vi "Demo_Main3.vi"() -> ()   [LabVIEW 2010]
uses:
  ControlCAN/ControlCAN.llb/DevType.ctl
  ControlCAN/ControlCAN.llb/CAN Channel.ctl
  ControlCAN/ControlCAN.llb/InitFlag.ctl
  ControlCAN/ControlCAN.llb/Mode.ctl
  ControlCAN/ControlCAN.llb/Fliter.ctl
  ControlCAN/ControlCAN.llb/VCI_CAN_OBJ.ctl
  ControlCAN/ControlCAN.llb/VCI_INIT_CONFIG.ctl
  ControlCAN/ControlCAN.llb/Return Val.ctl
  ControlCAN/ControlCAN.lvlib
panel:
  out "ERRO7":bool
  out "ERRO6":bool
  out "ERRO5":bool
  out "ERRO4":bool
  out "ERRO3":bool
  out "高温":bool
  out "高压":bool
  out "低压":bool
  out "warn7":bool
  out "warn6":bool
  out "warn5":bool
  out "warn4":bool
  out "warn3":bool
  out "高温":bool
  out "warn1":bool
  out "warn0":bool
  out "温度":dbl format="%#.6f"
  out "转速":dbl(graph)
  out "CAN ID":u8 format="%x"
  out "数组":u8[](array[numeric]) format="%x"
  in  "DATA_SAVE_W":bool
  out "CI_K0_回":u16
  out "BI_K0_回":u16
  in  "CI_K0_R":bool
  in  "BI_K0_R":bool
  in  "CI_K0_W":bool
  in  "BI_K0_W":bool
  in  "C电流零偏":u16
  in  "B电流零偏":u16
  in  "AI_K0_R":bool
  in  "A电流零偏":u16
  out "AI_K0_回":u16
  in  "AI_K0_W":bool
  out "Sin":i32
  out "Cosin":i32
  in  "加速度_R":bool
  in  "加速度":dbl min=0.0 max=8000.0 format="%#.6f"
  out "加速度_回":dbl format="%#.6f"
  in  "加速度_W":bool
  in  "速度环KI_R":bool
  in  "速度环KP_R":bool
  in  "速度环KI":dbl format="%#.6f"
  out "速度环KI_回":dbl format="%#.6f"
  in  "速度环KI_W":bool
  in  "速度环KP":dbl format="%#.6f"
  out "速度环KP_回":dbl format="%#.6f"
  in  "速度环KP_W":bool
  in  "电流环KI_R":bool
  in  "电流环KP_R":bool
  in  "电流环KI":dbl format="%#.6f"
  out "电流环KI_回":dbl format="%#.6f"
  in  "电流环KI_W":bool
  in  "电流环KP":dbl format="%#.6f"
  out "电流环KP_回":dbl format="%#.6f"
  in  "电流环KP_W":bool
  out "波形图表3":dbl(graph)
  out "波形图表2":dbl(graph)
  out "波形图表1":dbl(graph)
  out "sCnt":u32 caption="处理统计"
  out "模式_回":string(combo)="00"
  in  "模式_R":bool
  in  "设定电流_R":bool
  in  "设定位置_R":bool
  in  "设定速度_R":bool
  in  "存储路径":path
  in  "保存":bool
  out "保存_S":bool
  in  "模式_W":bool
  in  "模式":string(combo)="00"
  in  "设定电流":dbl format="%#.6f"
  out "设定电流_回":dbl format="%#.6f"
  in  "设定电流_W":bool
  in  "设定位置":dbl format="%#.6f"
  out "设定位置_回":dbl format="%#.6f"
  in  "设定位置_W":bool
  in  "设定速度":dbl format="%#.1f"
  out "设定速度_回":dbl format="%#.6f"
  in  "设定速度_W":bool
  in  "监测_W":bool
  in  "监测":string(combo)="30"
  out "电机ID_R":u32
  in  "Clear":bool
  out "Ualfa":dbl format="%#.6f"
  out "Ubate":dbl format="%#.6f"
  out "Uq":dbl format="%#.6f"
  out "Ud":dbl format="%#.6f"
  out "PWM1":u16
  out "PWM2":u16
  out "PWM3":u16
  out "sector":u8
  out "Iqnow":dbl
  out "Idnow":dbl
  out "Ialfa":dbl
  out "Ibeta":dbl
  out "A电流":dbl
  out "C电流":dbl
  out "B电流":dbl
  out "供电电压":dbl
  out "机械角度":dbl format="%.2f"
  out "电气角度":dbl
  out "转速":dbl
  out "CAN STD_ID":u32 format="%x"
  in  "电机ID":string(combo)="00"
  in  "电机ID_W":bool
  out "RecvCnt":u32 caption="接收统计"
  out "SendCnt":u32 caption="发送统计"
  in  "Format":u8(ring) items=["标准帧", "扩展帧"]
  in  "Type":u8(ring) items=["数据帧", "远程帧"]
  in  "Data":string="00 01 02 03 04 05 06 07"
  in  "ID":u32=291 format="0x%x"
  in  "Send":bool
  in  "RcvEnable":bool=TRUE
  out "Open":bool
  in  "Fliter":T1=1 items=["接收所有类型"=1, "只接收标准帧"=2, "只接收扩展帧"=3]
  in  "kBaudRate":u8(ring)=12 caption="波特率" items=["5k bps"=1, "10k bps"=2, "20k bps"=3, "40k bps"=4, "50k bps"=5, "80k bps"=6, "100k bps"=7, "125k bps"=8, "200k bps"=9, "250k bps"=10, "400k bps"=11, "500k bps"=12, "666k bps"=13, "800k bps"=14, "1000k bps"=15, "33.33k bps"=16, "66.66k bps"=17, "83.33k bps"=18]
  in  "Mode":T2 caption="工作模式" items=["正常工作", "仅侦听模式", "自测模式（环回）"]
  in  "InitFlag":T3 caption="初始化参数" items=["使用Flash参数", "使用界面设置参数"]
  in  "AccMask":u32=4294967295 caption="接收屏蔽码" format="%08x"
  in  "AccCode":u32 caption="接收过滤码" format="%08x"
  in  "Close":bool
  in  "Open":bool
  in  "Channel":T4 caption="CAN通道" items=["通道1", "通道2"]
  in  "DevType":T5=3 caption="设备类型" items=["USB-CAN"=2, "USB-CAN2"=3]
  # "."
  # "发送指令帧包"
  # "CAN\n  ID"
  # "DATA"
  # "DATA"
  # "DATA"
  # "0"
  # "1"
  # "7"
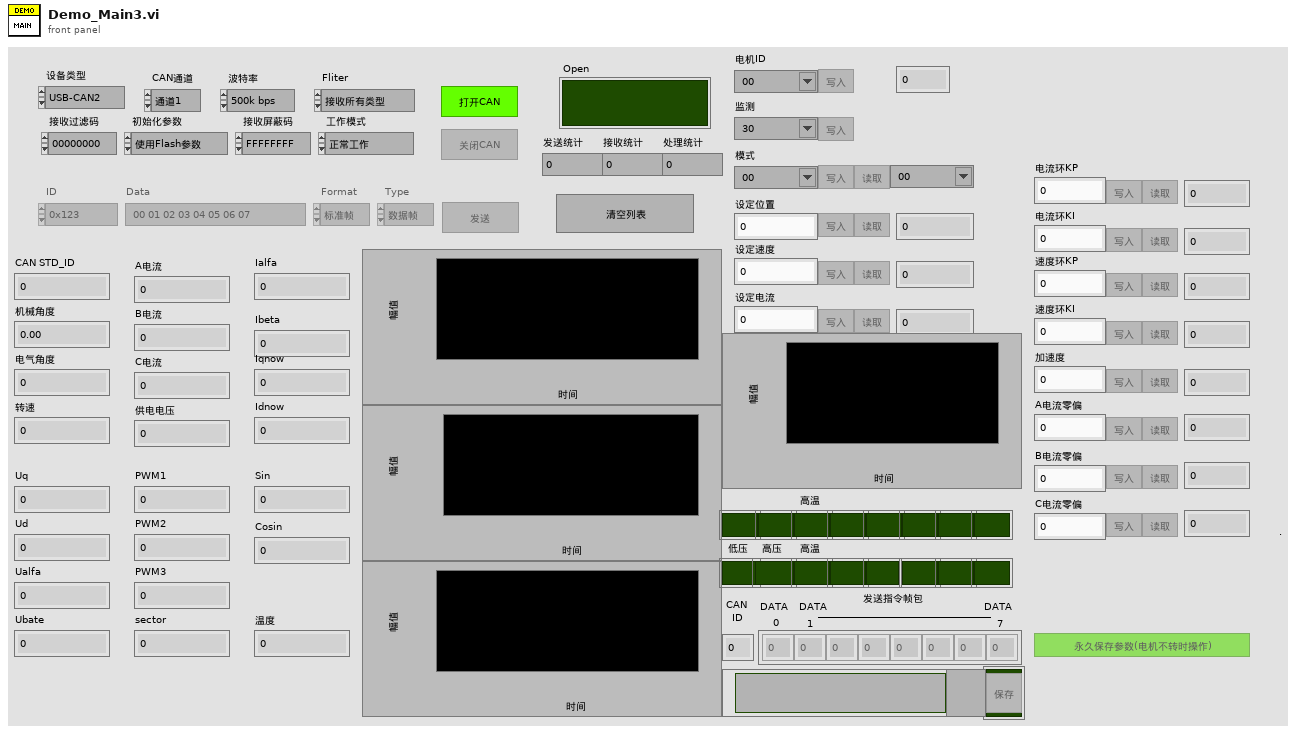
[diagram p1: front panel]
types:
  T1 = typedef "ControlCAN.lvlib/Fliter.ctl" = u8
  T2 = typedef "ControlCAN.lvlib/Mode.ctl" = u8
  T3 = typedef "ControlCAN.lvlib/InitFlag.ctl" = u32
  T4 = typedef "ControlCAN.lvlib/CAN Channel.ctl" = u32
  T5 = typedef "ControlCAN.lvlib/DevType.ctl" = u32
  T6 = typedef "ControlCAN.lvlib/VCI_CAN_OBJ.ctl" = cluster{"ID":u32, "TimeStamp":u32, "TimeFlag":u8, "SendType":u8, "RemoteFlag":u8, "ExternFlag":u8, "DataLen":u8, "Data":u8[], "Reserved":u8[]}
  T7 = cluster{"Type":enum16{"接收", "发送"}, "Channel":T4, "Time":timestamp, "VCI_CAN_OBJ":T6}[]
  T8 = typedef "ControlCAN.lvlib/VCI_INIT_CONFIG.ctl" = cluster{"AccCode":u32, "AccMask":u32, "InitFlag":T3, "Fliter":T1, "Timing0":u8, "Timing1":u8, "Mode":T2}
  T9 = cluster{"DevType":T5, "DevIndex":u32, "CanIndex":T4, "VCI_INIT_CONFIG":T8}
  T10 = typedef "ControlCAN.lvlib/Return Val.ctl" = i32
  T11 = enum16{"open", "replace", "create", "open or create", "replace or create", "replace or create with confirmation"}
  T12 = cluster{"[0]":cluster{"Type":enum16{"接收", "发送"}, "Channel":T4, "Time":timestamp, "VCI_CAN_OBJ":T6}}
  T13 = cluster{"Type":enum16{"接收", "发送"}, "Channel":T4, "Time":timestamp, "VCI_CAN_OBJ":T6}
  T14 = cluster{"Data[0]":u8, "Data[1]":u8, "Data[2]":u8, "Data[3]":u8, "Data[4]":u8, "Data[5]":u8, "Data[6]":u8, "Data[7]":u8}
  T15 = cluster{"Boolean array[0]":bool, "Boolean array[1]":bool, "Boolean array[2]":bool, "Boolean array[3]":bool, "Boolean array[4]":bool, "Boolean array[5]":bool, "Boolean array[6]":bool, "Boolean array[7]":bool}
  T16 = enum32{"invalid app kind", "Development System", "Run Time System", "Student Edition", "Embedded LabVIEW", "Evaluation", "Custom"}
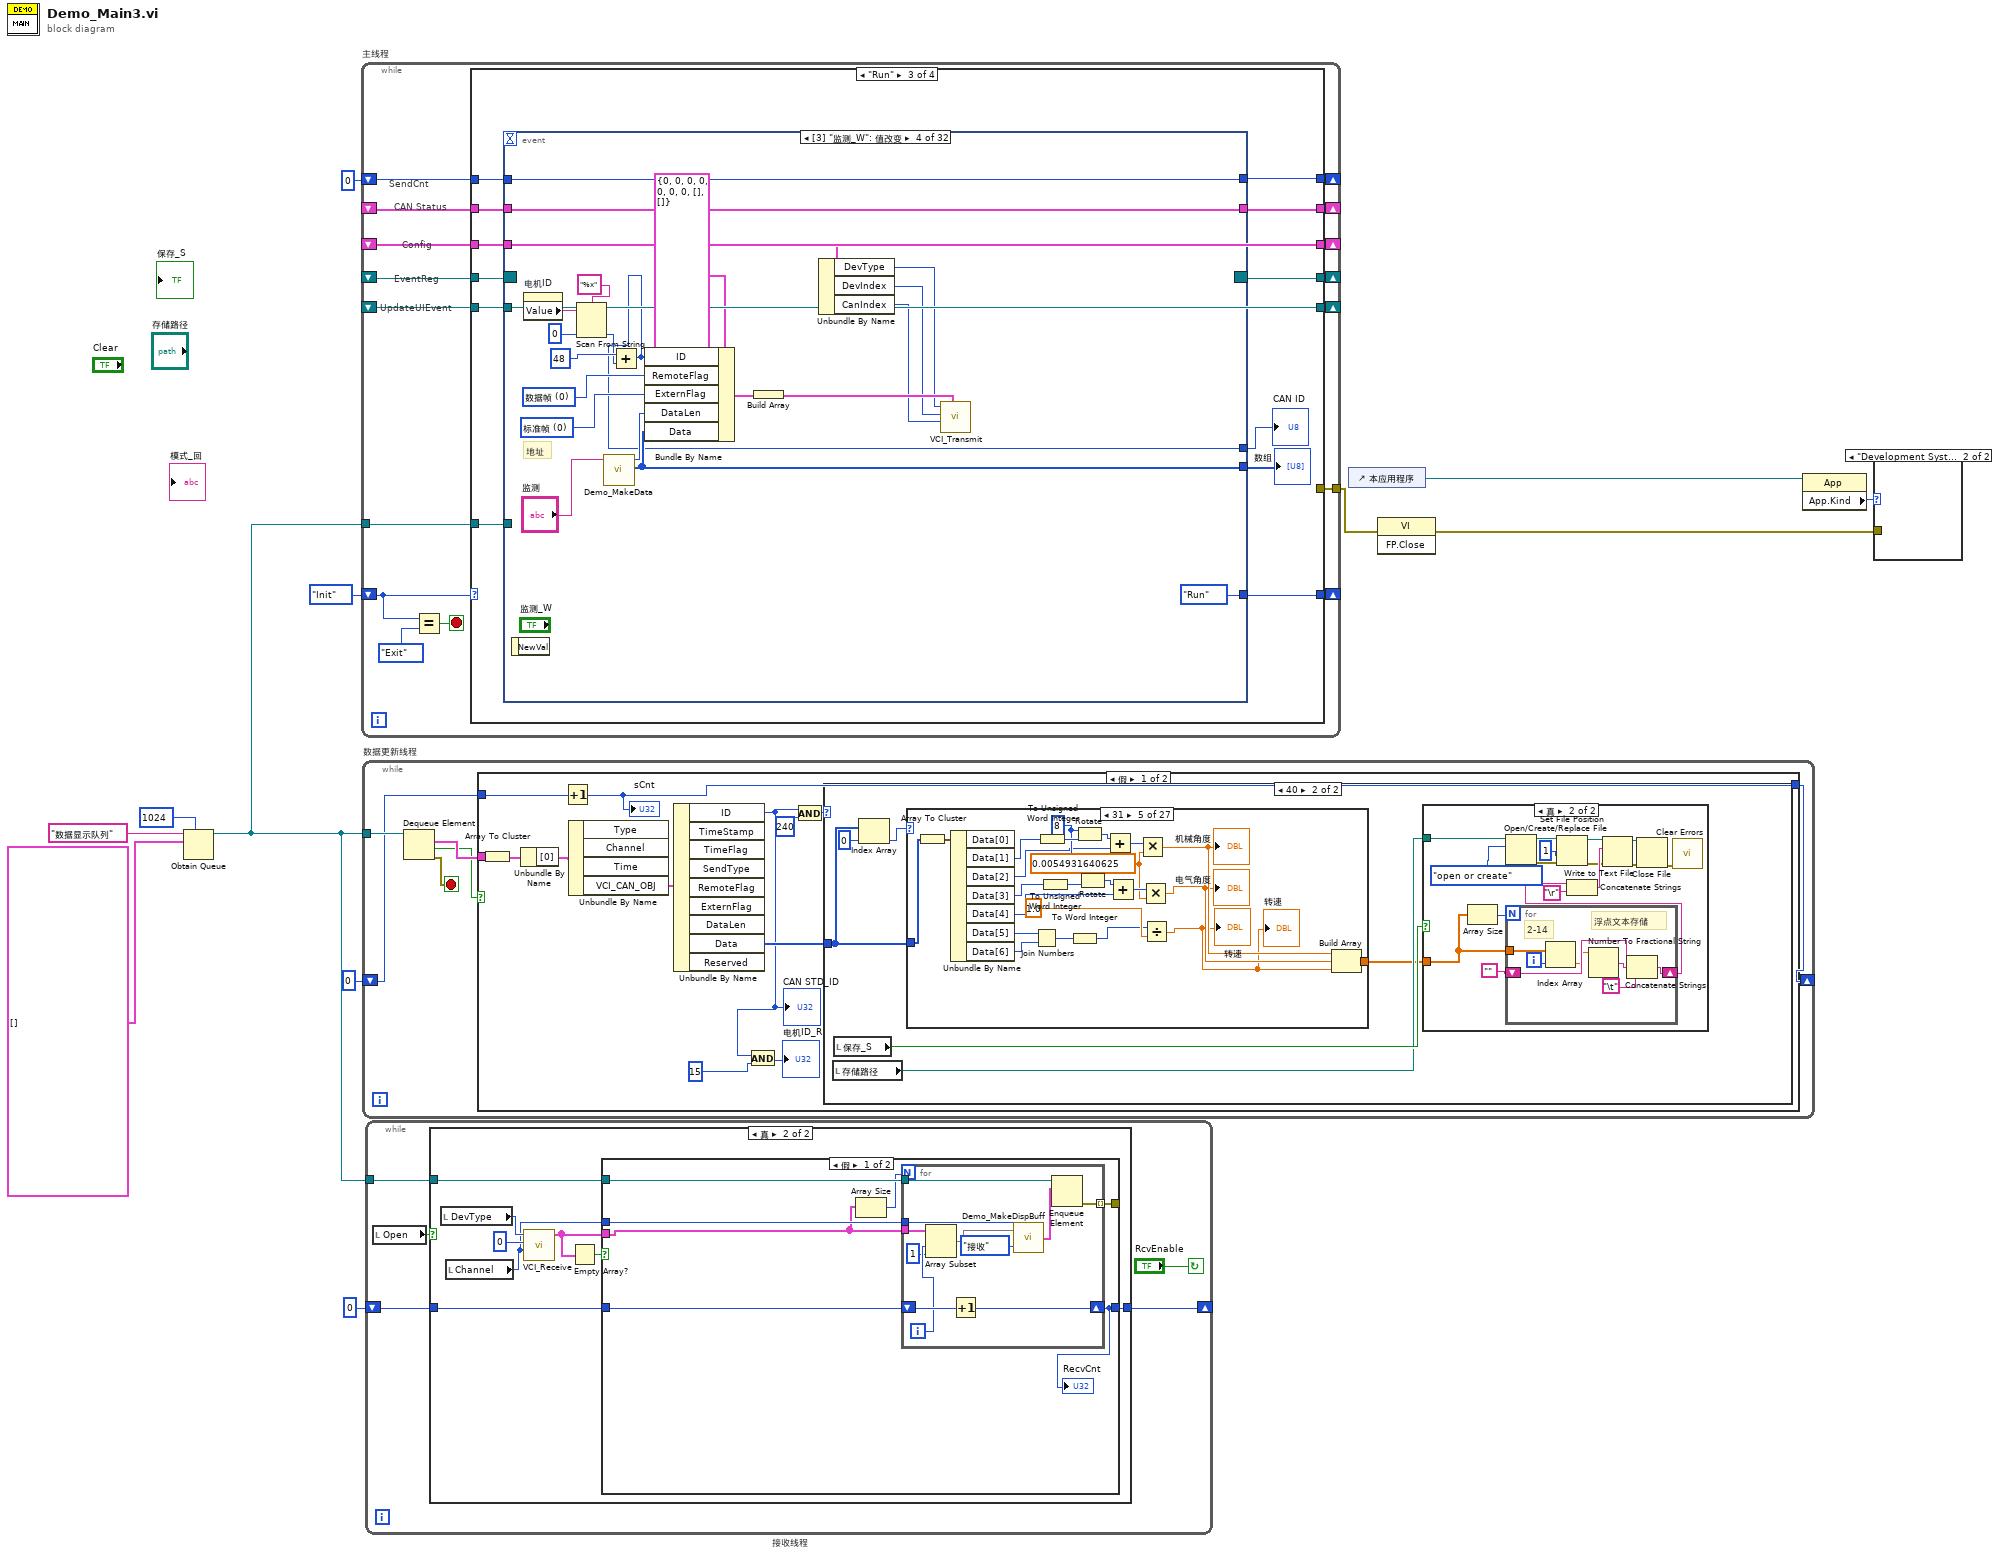
[diagram p0: block diagram]
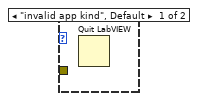
[diagram p2: hidden frame]
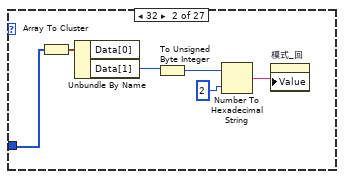
[diagram p6: hidden frame]
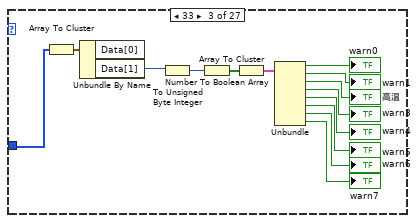
[diagram p7: hidden frame]
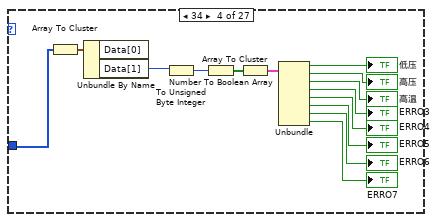
[diagram p8: hidden frame]
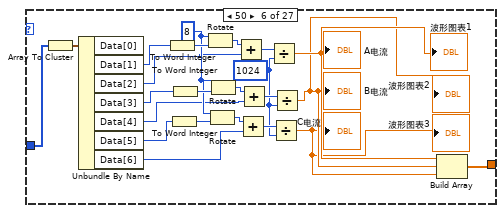
[diagram p9: hidden frame]
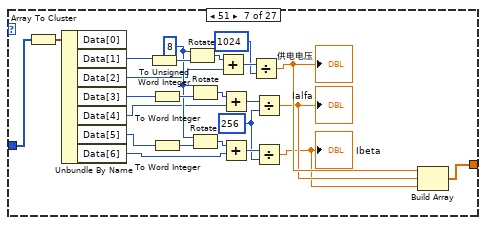
[diagram p10: hidden frame]
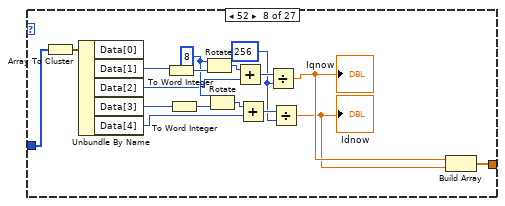
[diagram p11: hidden frame]
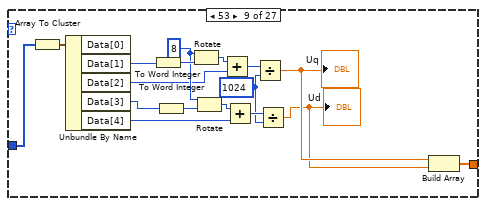
[diagram p12: hidden frame]
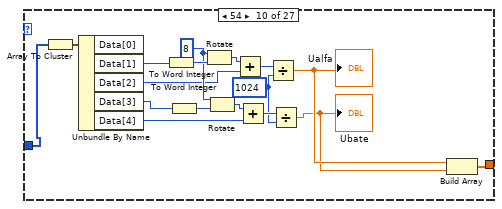
[diagram p13: hidden frame]
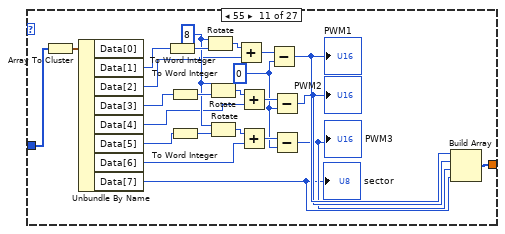
[diagram p14: hidden frame]
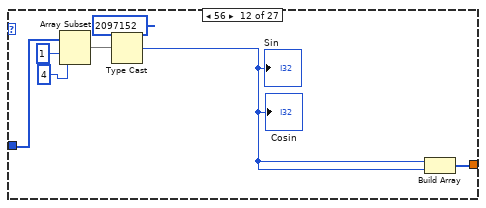
[diagram p15: hidden frame]
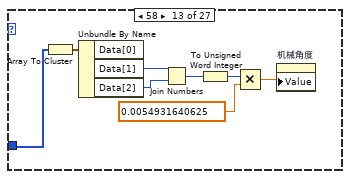
[diagram p16: hidden frame]
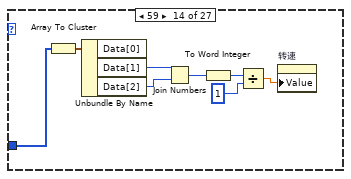
[diagram p17: hidden frame]
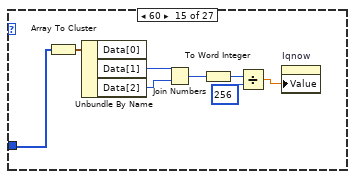
[diagram p18: hidden frame]
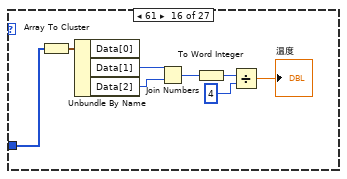
[diagram p19: hidden frame]
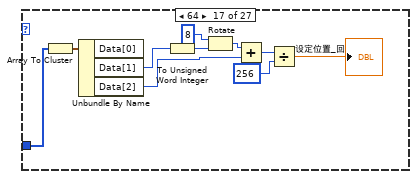
[diagram p20: hidden frame]
diagram:
  n1 = Obtain Queue(max queue size (-1, unlimited)=1024, name (unnamed)="数据显示队列" ("名称（未命名）"), element data type=T7 []) -> (queue out=w9:refnum<queue>)  [unwired: 2 in, 2 out]
  n2 = while "主线程" {
    shift-right: [w24] -> _
    shift-left: enum16{"Init", "Wait", "Run", "Exit"}."Init" -> [w27]
    shift-right: [w25] -> _
    shift-left: _ -> [w26]
    shift-right: [w23] -> _
    shift-left: _ -> [w22]
    tunnel: w9 -> [w21]
    shift-right: [w19] -> _
    shift-left: _ -> [w18]
    shift-right: [w17] -> _
    shift-left: _ -> [w16]
    shift-right: [w14] -> _
    shift-left: u32 0 -> [w15]
    tunnel: [w13] -> w4
    stop <- w28 stop-if-true
    # "CAN Status"
    # "Config"
    # "EventReg"
    # "UpdateUIEvent"
    # "SendCnt"
    n3 = Equal?(x=w27, y=enum16{"Init", "Wait", "Run", "Exit"}."Exit") -> (x = y?=w28:bool)
    n4 = case shown="\"Run\"" w27 {
      tunnel: w26 -> [_ w57 w158 w852]
      tunnel: [w48 w56 w157 w852] -> w25
      tunnel: [enum16{"Init", "Wait", "Run", "Exit"}."Wait" w53 w160 enum16{"Init", "Wait", "Run", "Exit"}."Exit"] -> w24
      tunnel: [w44 w54 w156 w850] -> w23
      tunnel: w22 -> [_ w55 w156 w850]
      tunnel: w21 -> [_ w52 w159 w856]
      tunnel: [w36 w51 w154 w855] -> w19
      tunnel: w18 -> [_ w51 w155 w855]
      tunnel: [w35 w50 w153 w853] -> w17
      tunnel: w16 -> [_ w50 w153 w853]
      tunnel: w15 -> [w33 w49 w152 w848]
      tunnel: [w33 w49 w151 w848] -> w14
      tunnel: [_ _ _ errorcluster {"status"=FALSE, "code"=0, "source"=""} ("error constant")] -> w13
      frame "Init", Default {
        w37 = cluster{"CANOpen":bool} {"CANOpen"=FALSE}  # UpdateUI
        w47 = T9 {"DevType"=2, "DevIndex"=0, "CanIndex"=0, "VCI_INIT_CONFIG"={"AccCode"=0, "AccMask"=0, "InitFlag"=0, "Fliter"=0, "Timing0"=0, "Timing1"=0, "Mode"=0}}  # Config
        w48 = cluster{"Open":bool, "SendCnt":u32} {"Open"=FALSE, "SendCnt"=0}  # CAN Status
        n5 = property class="VI"("Front Panel.Closeable"=TRUE ("前面板窗口:可关闭")) -> ()  [unwired: 2 in, 2 out]
        n6 = invoke class="VI" method="Default Vals.Reinit All"() -> ()  [unwired: 3 in, 3 out]
        n7 = call "Demo_GetT0T1.vi"("kBaudRate"="kBaudRate") -> ("Timing0"=w30:u8, "Timing1"=w29:u8)
        n8 = Bundle By Name(cluster=w47, "DevType"="DevType", "CanIndex"="Channel", "VCI_INIT_CONFIG.AccCode"="AccCode", "VCI_INIT_CONFIG.AccMask"="AccMask", "VCI_INIT_CONFIG.InitFlag"="InitFlag", "VCI_INIT_CONFIG.Fliter"="Fliter", "VCI_INIT_CONFIG.Timing0"=w30, "VCI_INIT_CONFIG.Timing1"=w29, "VCI_INIT_CONFIG.Mode"="Mode") -> (w44:T9)
        n9 = local write "RcvEnable"(TRUE ("RcvEnable")) -> ()
        n10 = Create User Event(user event datatype=w37) -> (user event=w35:refnum<user-event>)  [unwired: 1 in, 1 out]
        n11 = register-events(w35) -> (reference out=w36:refnum<event-registration>)  [unwired: 2 in, 1 out]
      }
      frame "Wait" {
        n12 = event shown="[0] \"Open\": 值改变" {
          selector: _ -> [_ _ _ _ _ _ _ _ _ _]
          dyn-events: _ -> [_ _ _ _ _ _ _ _ _ _]
          timeout: _ -> [_ _ _ _ _ _ _ _ _ _]
          tunnel: w57 -> [w61 w101 w111 w116 w121 w126 w131 w136 w143 w148]
          tunnel: [w60 w101 w111 w116 w121 w126 w131 w136 w143 w148] -> w56
          tunnel: w55 -> [w71 w100 w110 w115 w120 w125 w130 w135 w142 w147]
          tunnel: [w71 w100 w109 w113 w118 w123 w128 w133 w141 w145] -> w54
          tunnel: [w62 enum16{"Init", "Wait", "Run", "Exit"}."Exit" enum16{"Init", "Wait", "Run", "Exit"}."Wait" enum16{"Init", "Wait", "Run", "Exit"}."Wait" enum16{"Init", "Wait", "Run", "Exit"}."Wait" enum16{"Init", "Wait", "Run", "Exit"}."Wait" enum16{"Init", "Wait", "Run", "Exit"}."Wait" enum16{"Init", "Wait", "Run", "Exit"}."Wait" enum16{"Init", "Wait", "Run", "Exit"}."Wait" enum16{"Init", "Wait", "Run", "Exit"}."Wait"] -> w53
          tunnel: w52 -> [_ _ _ _ _ _ _ _ _ _]
          tunnel: w50 -> [w59 _ _ _ _ _ _ _ _ _]
          event "Open": Value Change {
            w65 = T10 1 items=["OK"=1, "ERROR1"=0, "ERROR2"=-1] ("y")
            # "打开CAN的步骤：\n1.Open\n2.Init\n3.Start"
            n13 = event-data() -> ()  [unwired: 2 out]
            n14 = Unbundle By Name(w71) -> ("DevType"=w70:T5, "DevIndex"=w69:u32)
            n15 = call "VCI_OpenDevice.vi"("DevIndex"=w69, "DevType"=w70) -> ("error out"=w66:errorcluster, "Return Val"=w68:T10)  [unwired: 2 in, 6 out]
            n16 = Equal?(x=w68, y=w65) -> (x = y?=w67:bool)
            n17 = case shown="真" w67 {
              tunnel: w66 -> [_ w86]
              tunnel: w71 -> [_ w85]
              tunnel: w65 -> [_ w77]
              tunnel: [_ w76] -> w58
              frame False {
              }
              frame True {
                n18 = Unbundle By Name(w85) -> ("VCI_INIT_CONFIG"=w84:T8, "DevType"=w80:T5, "DevIndex"=w79:u32, "CanIndex"=w78:T4)
                n19 = call "VCI_InitCAN.vi"("VCI_INIT_CONFIG"=w84, "error in (no error)"=w86, "CANIndex"=w78, "DevIndex"=w79, "DevType"=w80) -> ("error out"=w81:errorcluster, "Return Val"=w83:T10)  [unwired: 5 out]
                n20 = Equal?(x=w77, y=w83) -> (x = y?=w82:bool)
                n21 = case shown="真" w82 {
                  tunnel: w81 -> [_ w97]
                  tunnel: w80 -> [_ w96]
                  tunnel: w79 -> [_ w95]
                  tunnel: w78 -> [_ w94]
                  tunnel: w77 -> [_ w92]
                  tunnel: [_ w88] -> w76
                  frame False {
                  }
                  frame True {
                    n22 = call "VCI_StartCAN.vi"("error in (no error)"=w97, "CANIndex"=w94, "DevIndex"=w95, "DevType"=w96) -> ("error out"=w90:errorcluster, "Return Val"=w93:T10)  [unwired: 6 out]
                    n23 = Unbundle By Name(w90) -> ("status"=w87:bool)
                    n24 = Equal?(x=w92, y=w93) -> (x = y?=w91:bool)
                    n25 = Not(x=w87) -> (.not. x?=w89:bool)
                    n26 = And(x=w91, y=w89) -> (x .and. y?=w88:bool)
                  }
                }
              }
            }
            n27 = case shown="真" w58 {
              tunnel: w59 -> [_ w75]
              tunnel: w58 -> [_ w73]
              frame False {
              }
              frame True {
                n28 = Bundle By Name(cluster=cluster{"CANOpen":bool} {"CANOpen"=FALSE} ("事件数据"), "CANOpen"=w73) -> (w72:cluster{"CANOpen":bool})
                n29 = Generate User Event(user event=w75, event data cluster=w72) -> ()  [unwired: 1 in, 2 out]
              }
            }
            n30 = Select(t=enum16{"Init", "Wait", "Run", "Exit"}."Run", s=w58, f=enum16{"Init", "Wait", "Run", "Exit"}."Wait") -> (s? t:f=w62:enum16{"Init", "Wait", "Run", "Exit"})
            n31 = Bundle By Name(cluster=w61, "Open"=w58) -> (w60:cluster{"Open":bool, "SendCnt":u32})
          }
          event Panel Close? {
            n32 = event-data() -> ()  [unwired: 2 out]
            n33 = event-data("Discard?"=TRUE ("放弃？")) -> ()  [unwired: 1 in, 1 out]
          }
          event Value Change {
            w107 = T5 3 items=["USB-CAN"=2, "USB-CAN2"=3] ("y")
            n34 = event-data() -> ("NewVal"=w108:T5)  [unwired: 1 out]
            n35 = Equal?(x=w108, y=w107) -> (x = y?=w106:bool)
            n36 = Bundle By Name(cluster=w110, "DevType"=w108) -> (w109:T9)
            n37 = Select(t=i32[] [] ("禁用项[]"), s=w106, f=i32[] [1] ("禁用项[]")) -> (s? t:f=w105:i32[])
            n38 = property on="Channel" class="Ring (严格)"("Disabled Items []"=w105) -> ()  [unwired: 2 in, 2 out]
          }
          event Value Change {
            n39 = event-data() -> ("NewVal"=w114:T4)  [unwired: 1 out]
            n40 = Bundle By Name(cluster=w115, "CanIndex"=w114) -> (w113:T9)
          }
          event "AccCode": Value Change {
            n41 = event-data() -> ("NewVal"=w119:u32)  [unwired: 1 out]
            n42 = Bundle By Name(cluster=w120, "VCI_INIT_CONFIG.AccCode"=w119) -> (w118:T9)
          }
          event "AccMask": Value Change {
            n43 = event-data() -> ("NewVal"=w124:u32)  [unwired: 1 out]
            n44 = Bundle By Name(cluster=w125, "VCI_INIT_CONFIG.AccMask"=w124) -> (w123:T9)
          }
          event Value Change {
            n45 = event-data() -> ("NewVal"=w129:T3)  [unwired: 1 out]
            n46 = Bundle By Name(cluster=w130, "VCI_INIT_CONFIG.InitFlag"=w129) -> (w128:T9)
          }
          event Value Change {
            n47 = event-data() -> ("NewVal"=w134:T2)  [unwired: 1 out]
            n48 = Bundle By Name(cluster=w135, "VCI_INIT_CONFIG.Mode"=w134) -> (w133:T9)
          }
          event "kBaudRate": Value Change {
            n49 = event-data() -> ("NewVal"=w139:u8)  [unwired: 1 out]
            n50 = call "Demo_GetT0T1.vi"("kBaudRate"=w139) -> ("Timing0"=w138:u8, "Timing1"=w137:u8)
            n51 = Bundle By Name(cluster=w142, "VCI_INIT_CONFIG.Timing0"=w138, "VCI_INIT_CONFIG.Timing1"=w137) -> (w141:T9)
          }
          event Value Change {
            n52 = event-data() -> ("NewVal"=w146:T1)  [unwired: 1 out]
            n53 = Bundle By Name(cluster=w147, "VCI_INIT_CONFIG.Fliter"=w146) -> (w145:T9)
          }
        }
      }
      frame "Run" {
        n54 = event shown="[3] \"监测_W\": 值改变" {
          selector: w155 -> [_ _ _ _ _ _ _ _ _ _ _ _ _ _ _ _ _ _ _ _ _ _ _ _ _ _ _ _ _ _ _ _]
          dyn-events: [_ _ _ _ _ _ _ _ _ _ _ _ _ _ _ _ _ _ _ _ _ _ _ _ _ _ _ _ _ _ _ _] -> w154
          timeout: _ -> [_ _ _ _ _ _ _ _ _ _ _ _ _ _ _ _ _ _ _ _ _ _ _ _ _ _ _ _ _ _ _ _]
          tunnel: [enum16{"Init", "Wait", "Run", "Exit"}."Run" enum16{"Init", "Wait", "Run", "Exit"}."Run" enum16{"Init", "Wait", "Run", "Exit"}."Run" enum16{"Init", "Wait", "Run", "Exit"}."Run" enum16{"Init", "Wait", "Run", "Exit"}."Run" enum16{"Init", "Wait", "Run", "Exit"}."Run" enum16{"Init", "Wait", "Run", "Exit"}."Run" enum16{"Init", "Wait", "Run", "Exit"}."Run" enum16{"Init", "Wait", "Run", "Exit"}."Run" enum16{"Init", "Wait", "Run", "Exit"}."Run" enum16{"Init", "Wait", "Run", "Exit"}."Run" enum16{"Init", "Wait", "Run", "Exit"}."Run" enum16{"Init", "Wait", "Run", "Exit"}."Run" enum16{"Init", "Wait", "Run", "Exit"}."Run" enum16{"Init", "Wait", "Run", "Exit"}."Run" enum16{"Init", "Wait", "Run", "Exit"}."Run" enum16{"Init", "Wait", "Run", "Exit"}."Run" enum16{"Init", "Wait", "Run", "Exit"}."Run" enum16{"Init", "Wait", "Run", "Exit"}."Run" enum16{"Init", "Wait", "Run", "Exit"}."Run" enum16{"Init", "Wait", "Run", "Exit"}."Run" enum16{"Init", "Wait", "Run", "Exit"}."Run" enum16{"Init", "Wait", "Run", "Exit"}."Run" enum16{"Init", "Wait", "Run", "Exit"}."Run" enum16{"Init", "Wait", "Run", "Exit"}."Run" enum16{"Init", "Wait", "Run", "Exit"}."Run" enum16{"Init", "Wait", "Run", "Exit"}."Run" enum16{"Init", "Wait", "Run", "Exit"}."Run" enum16{"Init", "Wait", "Run", "Exit"}."Run" enum16{"Init", "Wait", "Run", "Exit"}."Run" enum16{"Init", "Wait", "Run", "Exit"}."Run" w840] -> w160
          tunnel: w159 -> [_ _ _ _ _ _ _ _ _ _ _ _ _ _ _ _ _ _ _ _ _ _ _ _ _ _ _ _ _ _ _ _]
          tunnel: [w162 w179 w196 w217 w240 w261 w287 w313 w339 w365 w391 w417 w443 w469 w493 w517 w541 w562 w583 w604 w625 w646 w667 w688 w709 w730 w751 w772 w793 w821 w827 w846] -> w157
          tunnel: w158 -> [w162 w179 w196 w217 w240 w261 w287 w313 w339 w365 w391 w417 w443 w469 w493 w517 w541 w562 w583 w604 w625 w646 w667 w688 w709 w730 w751 w772 w793 w821 w829 w846]
          tunnel: w156 -> [_ w174 w186 w206 w222 w244 w272 w295 w321 w344 w370 w396 w422 w448 w474 w498 w522 w545 w566 w587 w608 w629 w650 w671 w692 w713 w734 w755 w776 _ w834 _]
          tunnel: w153 -> [_ _ _ _ _ _ _ _ _ _ _ _ _ _ _ _ _ _ _ _ _ _ _ _ _ _ _ _ _ _ w826 _]
          tunnel: w152 -> [w161 w167 w195 w216 w239 w260 w286 w312 w338 w364 w390 w416 w442 w468 w492 w516 w540 w561 w582 w603 w624 w645 w666 w687 w708 w729 w750 w771 w792 w820 w822 w839]
          tunnel: [w161 w166 w195 w216 w239 w260 w286 w312 w338 w364 w390 w416 w442 w468 w492 w516 w540 w561 w582 w603 w624 w645 w666 w687 w708 w729 w750 w771 w792 w820 w822 w839] -> w151
          tunnel: [_ _ w182 w198 w220 w242 w263 w289 w315 w341 w367 w393 w419 w445 w471 w495 w519 w543 w564 w585 w606 w627 w648 w669 w690 w711 w732 w753 w774 _ _ _] -> w150
          tunnel: [_ _ w181 w197 w219 w241 w262 w288 w314 w340 w366 w392 w418 w444 w470 w494 w518 w542 w563 w584 w605 w626 w647 w668 w689 w710 w731 w752 w773 _ _ _] -> w149
          event Timeout {
            n55 = event-data() -> ()  [unwired: 3 out]
          }
          event "Send": Value Change {
            n56 = event-data() -> ()  [unwired: 2 out]
            n57 = Increment(x=w167) -> (x+1=w166:u32)
            "SendCnt" <- w166
            n58 = call "Demo_MakeData.vi"("DataString"="Data") -> ("Data"=w169:u8[], "DataLen"=w170:u8)  [unwired: 9 out]
            n59 = Bundle By Name(cluster=T6 {"ID"=0, "TimeStamp"=0, "TimeFlag"=0, "SendType"=0, "RemoteFlag"=0, "ExternFlag"=0, "DataLen"=0, "Data"=[], "Reserved"=[]} ("Send"), "ID"="ID", "RemoteFlag"="Type", "ExternFlag"="Format", "DataLen"=w170, "Data"=w169) -> (w164:T6)
            n60 = Build Array(w164) -> (w165:T6[])
            n61 = Unbundle By Name(w174) -> ("DevType"=w173:T5, "DevIndex"=w172:u32, "CanIndex"=w168:T4)
            n62 = call "VCI_Transmit.vi"("Buffer"=w165, "CANIndex"=w168, "DevIndex"=w172, "DevType"=w173) -> ()  [unwired: 1 in, 7 out]
          }
          event "电机ID_W": Value Change {
            w185 = u8 0 items=["数据帧", "遥控帧"]
            w181 = u32 138
            w184 = u8 0 items=["标准帧", "扩展帧"]
            n63 = event-data() -> ()  [unwired: 2 out]
            n64 = call "Demo_MakeData.vi"("DataString"="电机ID") -> ("Data"=w182:u8[], "DataLen"=w190:u8)  [unwired: 9 out]
            n65 = Bundle By Name(cluster=T6 {"ID"=0, "TimeStamp"=0, "TimeFlag"=0, "SendType"=0, "RemoteFlag"=0, "ExternFlag"=0, "DataLen"=0, "Data"=[], "Reserved"=[]} ("Send"), "ID"=w181, "RemoteFlag"=w185, "ExternFlag"=w184, "DataLen"=w190, "Data"=w182) -> (w187:T6)
            n66 = Build Array(w187) -> (w188:T6[])
            n67 = Unbundle By Name(w186) -> ("DevType"=w192:T5, "DevIndex"=w191:u32, "CanIndex"=w189:T4)
            n68 = call "VCI_Transmit.vi"("Buffer"=w188, "CANIndex"=w189, "DevIndex"=w191, "DevType"=w192) -> ()  [unwired: 1 in, 7 out]
          }
          event "监测_W": Value Change {
            w214 = u8 0 items=["数据帧", "遥控帧"]
            w215 = u8 0 items=["标准帧", "扩展帧"]
            # "地址"
            n69 = event-data() -> ()  [unwired: 2 out]
            n70 = property on="电机ID" class="CmbBox"() -> ("Value"=w203:string)  [unwired: 2 in, 2 out]
            n71 = Scan From String(format string="%x" ("格式字符串"), input string=w203, default 1=u8 0) -> (output 1=w200:u8)  [unwired: 2 in, 3 out]
            n72 = call "Demo_MakeData.vi"("DataString"="监测") -> ("Data"=w198:u8[], "DataLen"=w210:u8)  [unwired: 9 out]
            n73 = Add(x=u32 48, y=w200) -> (x+y=w197:u32)
            n74 = Bundle By Name(cluster=T6 {"ID"=0, "TimeStamp"=0, "TimeFlag"=0, "SendType"=0, "RemoteFlag"=0, "ExternFlag"=0, "DataLen"=0, "Data"=[], "Reserved"=[]} ("Send"), "ID"=w197, "RemoteFlag"=w214, "ExternFlag"=w215, "DataLen"=w210, "Data"=w198) -> (w213:T6)
            n75 = Build Array(w213) -> (w212:T6[])
            n76 = Unbundle By Name(w206) -> ("DevType"=w208:T5, "DevIndex"=w209:u32, "CanIndex"=w211:T4)
            n77 = call "VCI_Transmit.vi"("Buffer"=w212, "CANIndex"=w211, "DevIndex"=w209, "DevType"=w208) -> ()  [unwired: 1 in, 7 out]
          }
          event "模式_W": Value Change {
            w224 = u8 0 items=["数据帧", "遥控帧"]
            w223 = u8 0 items=["标准帧", "扩展帧"]
            # "地址"
            n78 = event-data() -> ()  [unwired: 2 out]
            n79 = property on="电机ID" class="CmbBox"() -> ("Value"=w233:string)  [unwired: 2 in, 2 out]
            n80 = Concatenate Strings("20 ", "模式") -> (w237:string)
            n81 = Scan From String(format string="%x" ("格式字符串"), input string=w233, default 1=u8 0) -> (output 1=w236:u8)  [unwired: 2 in, 3 out]
            n82 = property on="模式_回" class="CmbBox"("Value"="模式") -> ()  [unwired: 2 in, 2 out]
            n83 = call "Demo_MakeData.vi"("DataString"=w237) -> ("Data"=w220:u8[], "DataLen"=w228:u8)  [unwired: 9 out]
            n84 = Add(x=u32 16, y=w236) -> (x+y=w219:u32)
            n85 = Bundle By Name(cluster=T6 {"ID"=0, "TimeStamp"=0, "TimeFlag"=0, "SendType"=0, "RemoteFlag"=0, "ExternFlag"=0, "DataLen"=0, "Data"=[], "Reserved"=[]} ("Send"), "ID"=w219, "RemoteFlag"=w224, "ExternFlag"=w223, "DataLen"=w228, "Data"=w220) -> (w225:T6)
            n86 = Build Array(w225) -> (w226:T6[])
            n87 = Unbundle By Name(w222) -> ("DevType"=w230:T5, "DevIndex"=w229:u32, "CanIndex"=w227:T4)
            n88 = call "VCI_Transmit.vi"("Buffer"=w226, "CANIndex"=w227, "DevIndex"=w229, "DevType"=w230) -> ()  [unwired: 1 in, 7 out]
          }
          event "模式_R": Value Change {
            w257 = u8 0 items=["数据帧", "遥控帧"]
            w258 = u8 0 items=["标准帧", "扩展帧"]
            # "地址"
            n89 = event-data() -> ()  [unwired: 2 out]
            n90 = property on="电机ID" class="CmbBox"() -> ("Value"=w248:string)  [unwired: 2 in, 2 out]
            n91 = Scan From String(format string="%x" ("格式字符串"), input string=w248, default 1=u8 0) -> (output 1=w245:u8)  [unwired: 2 in, 3 out]
            n92 = call "Demo_MakeData.vi"("DataString"="20 ") -> ("Data"=w242:u8[], "DataLen"=w253:u8)  [unwired: 9 out]
            n93 = Add(x=u32 48, y=w245) -> (x+y=w241:u32)
            n94 = Bundle By Name(cluster=T6 {"ID"=0, "TimeStamp"=0, "TimeFlag"=0, "SendType"=0, "RemoteFlag"=0, "ExternFlag"=0, "DataLen"=0, "Data"=[], "Reserved"=[]} ("Send"), "ID"=w241, "RemoteFlag"=w257, "ExternFlag"=w258, "DataLen"=w253, "Data"=w242) -> (w256:T6)
            n95 = Build Array(w256) -> (w255:T6[])
            n96 = Unbundle By Name(w244) -> ("DevType"=w251:T5, "DevIndex"=w252:u32, "CanIndex"=w254:T4)
            n97 = call "VCI_Transmit.vi"("Buffer"=w255, "CANIndex"=w254, "DevIndex"=w252, "DevType"=w251) -> ()  [unwired: 1 in, 7 out]
          }
          event "设定位置_W": Value Change {
            w274 = u8 0 items=["数据帧", "遥控帧"]
            w273 = u8 0 items=["标准帧", "扩展帧"]
            # "索引地址"
            n98 = event-data() -> ()  [unwired: 2 out]
            n99 = property on="电机ID" class="CmbBox"() -> ("Value"=w282:string)  [unwired: 2 in, 2 out]
            n100 = Multiply ("乘")(x="设定位置", y=u16 256) -> (x*y=w266:i16)
            n101 = Scan From String(format string="%x" ("格式字符串"), input string=w282, default 1=u8 0) -> (output 1=w285:u8)  [unwired: 2 in, 3 out]
            n102 = Split Number(x=w266) -> (hi(x)=w265:u8, lo(x)=w264:u8)
            n103 = Add(x=u32 16, y=w285) -> (x+y=w262:u32)
            n104 = Build Array(u8 64, w265, w264) -> (w263:u8[])
            n105 = Bundle By Name(cluster=T6 {"ID"=0, "TimeStamp"=0, "TimeFlag"=0, "SendType"=0, "RemoteFlag"=0, "ExternFlag"=0, "DataLen"=0, "Data"=[], "Reserved"=[]} ("Send"), "ID"=w262, "RemoteFlag"=w274, "ExternFlag"=w273, "DataLen"=u8 3, "Data"=w263) -> (w275:T6)
            n106 = Build Array(w275) -> (w276:T6[])
            n107 = Unbundle By Name(w272) -> ("DevType"=w279:T5, "DevIndex"=w278:u32, "CanIndex"=w277:T4)
            n108 = call "VCI_Transmit.vi"("Buffer"=w276, "CANIndex"=w277, "DevIndex"=w278, "DevType"=w279) -> ()  [unwired: 1 in, 7 out]
          }
          event "设定速度_W": Value Change {
            w307 = u8 0 items=["数据帧", "遥控帧"]
            w308 = u8 0 items=["标准帧", "扩展帧"]
            # "索引地址"
            n109 = event-data() -> ()  [unwired: 2 out]
            n110 = property on="电机ID" class="CmbBox"() -> ("Value"=w299:string)  [unwired: 2 in, 2 out]
            n111 = Multiply ("乘")(x="设定速度", y=i16 1) -> (x*y=w292:i16)
            n112 = Scan From String(format string="%x" ("格式字符串"), input string=w299, default 1=u8 0) -> (output 1=w296:u8)  [unwired: 2 in, 3 out]
            n113 = Split Number(x=w292) -> (hi(x)=w291:u8, lo(x)=w290:u8)
            n114 = Add(x=u32 16, y=w296) -> (x+y=w288:u32)
            n115 = Build Array(u8 65, w291, w290) -> (w289:u8[])
            n116 = Bundle By Name(cluster=T6 {"ID"=0, "TimeStamp"=0, "TimeFlag"=0, "SendType"=0, "RemoteFlag"=0, "ExternFlag"=0, "DataLen"=0, "Data"=[], "Reserved"=[]} ("Send"), "ID"=w288, "RemoteFlag"=w307, "ExternFlag"=w308, "DataLen"=u8 3, "Data"=w289) -> (w306:T6)
            n117 = Build Array(w306) -> (w305:T6[])
            n118 = Unbundle By Name(w295) -> ("DevType"=w302:T5, "DevIndex"=w303:u32, "CanIndex"=w304:T4)
            n119 = call "VCI_Transmit.vi"("Buffer"=w305, "CANIndex"=w304, "DevIndex"=w303, "DevType"=w302) -> ()  [unwired: 1 in, 7 out]
          }
          event "设定电流_W": Value Change {
            w326 = u8 0 items=["数据帧", "遥控帧"]
            w325 = u8 0 items=["标准帧", "扩展帧"]
            # "索引地址"
            n120 = event-data() -> ()  [unwired: 2 out]
            n121 = property on="电机ID" class="CmbBox"() -> ("Value"=w334:string)  [unwired: 2 in, 2 out]
            n122 = Multiply ("乘")(x="设定电流", y=i16 256) -> (x*y=w318:i16)
            n123 = Scan From String(format string="%x" ("格式字符串"), input string=w334, default 1=u8 0) -> (output 1=w337:u8)  [unwired: 2 in, 3 out]
            n124 = Split Number(x=w318) -> (hi(x)=w317:u8, lo(x)=w316:u8)
            n125 = Add(x=u32 16, y=w337) -> (x+y=w314:u32)
            n126 = Build Array(u8 66, w317, w316) -> (w315:u8[])
            n127 = Bundle By Name(cluster=T6 {"ID"=0, "TimeStamp"=0, "TimeFlag"=0, "SendType"=0, "RemoteFlag"=0, "ExternFlag"=0, "DataLen"=0, "Data"=[], "Reserved"=[]} ("Send"), "ID"=w314, "RemoteFlag"=w326, "ExternFlag"=w325, "DataLen"=u8 3, "Data"=w315) -> (w327:T6)
            n128 = Build Array(w327) -> (w328:T6[])
            n129 = Unbundle By Name(w321) -> ("DevType"=w331:T5, "DevIndex"=w330:u32, "CanIndex"=w329:T4)
            n130 = call "VCI_Transmit.vi"("Buffer"=w328, "CANIndex"=w329, "DevIndex"=w330, "DevType"=w331) -> ()  [unwired: 1 in, 7 out]
          }
          event "电流环KP_W": Value Change {
            w356 = u8 0 items=["数据帧", "遥控帧"]
            w357 = u8 0 items=["标准帧", "扩展帧"]
            # "索引地址"
            n131 = event-data() -> ()  [unwired: 2 out]
            n132 = property on="电机ID" class="CmbBox"() -> ("Value"=w348:string)  [unwired: 2 in, 2 out]
            n133 = Multiply ("乘")(x="电流环KP", y=u16 256) -> (x*y=w361:u16)
            n134 = Scan From String(format string="%x" ("格式字符串"), input string=w348, default 1=u8 0) -> (output 1=w345:u8)  [unwired: 2 in, 3 out]
            n135 = Split Number(x=w361) -> (hi(x)=w362:u8, lo(x)=w363:u8)
            n136 = Add(x=u32 16, y=w345) -> (x+y=w340:u32)
            n137 = Build Array(u8 81, w362, w363) -> (w341:u8[])
            n138 = Bundle By Name(cluster=T6 {"ID"=0, "TimeStamp"=0, "TimeFlag"=0, "SendType"=0, "RemoteFlag"=0, "ExternFlag"=0, "DataLen"=0, "Data"=[], "Reserved"=[]} ("Send"), "ID"=w340, "RemoteFlag"=w356, "ExternFlag"=w357, "DataLen"=u8 3, "Data"=w341) -> (w355:T6)
            n139 = Build Array(w355) -> (w354:T6[])
            n140 = Unbundle By Name(w344) -> ("DevType"=w351:T5, "DevIndex"=w352:u32, "CanIndex"=w353:T4)
            n141 = call "VCI_Transmit.vi"("Buffer"=w354, "CANIndex"=w353, "DevIndex"=w352, "DevType"=w351) -> ()  [unwired: 1 in, 7 out]
          }
          event "电流环KI_W": Value Change {
            w378 = u8 0 items=["数据帧", "遥控帧"]
            w377 = u8 0 items=["标准帧", "扩展帧"]
            # "索引地址"
            n142 = event-data() -> ()  [unwired: 2 out]
            n143 = property on="电机ID" class="CmbBox"() -> ("Value"=w386:string)  [unwired: 2 in, 2 out]
            n144 = Multiply ("乘")(x="电流环KI", y=u16 256) -> (x*y=w373:u16)
            n145 = Scan From String(format string="%x" ("格式字符串"), input string=w386, default 1=u8 0) -> (output 1=w389:u8)  [unwired: 2 in, 3 out]
            n146 = Split Number(x=w373) -> (hi(x)=w372:u8, lo(x)=w371:u8)
            n147 = Add(x=u32 16, y=w389) -> (x+y=w366:u32)
            n148 = Build Array(u8 82, w372, w371) -> (w367:u8[])
            n149 = Bundle By Name(cluster=T6 {"ID"=0, "TimeStamp"=0, "TimeFlag"=0, "SendType"=0, "RemoteFlag"=0, "ExternFlag"=0, "DataLen"=0, "Data"=[], "Reserved"=[]} ("Send"), "ID"=w366, "RemoteFlag"=w378, "ExternFlag"=w377, "DataLen"=u8 3, "Data"=w367) -> (w379:T6)
            n150 = Build Array(w379) -> (w380:T6[])
            n151 = Unbundle By Name(w370) -> ("DevType"=w383:T5, "DevIndex"=w382:u32, "CanIndex"=w381:T4)
            n152 = call "VCI_Transmit.vi"("Buffer"=w380, "CANIndex"=w381, "DevIndex"=w382, "DevType"=w383) -> ()  [unwired: 1 in, 7 out]
          }
          event "速度环KP_W": Value Change {
            w404 = u8 0 items=["数据帧", "遥控帧"]
            w403 = u8 0 items=["标准帧", "扩展帧"]
            # "索引地址"
            n153 = event-data() -> ()  [unwired: 2 out]
            n154 = property on="电机ID" class="CmbBox"() -> ("Value"=w412:string)  [unwired: 2 in, 2 out]
            n155 = Multiply ("乘")(x="速度环KP", y=u16 256) -> (x*y=w399:u16)
            n156 = Scan From String(format string="%x" ("格式字符串"), input string=w412, default 1=u8 0) -> (output 1=w415:u8)  [unwired: 2 in, 3 out]
            n157 = Split Number(x=w399) -> (hi(x)=w398:u8, lo(x)=w397:u8)
            n158 = Add(x=u32 16, y=w415) -> (x+y=w392:u32)
            n159 = Build Array(u8 83, w398, w397) -> (w393:u8[])
            n160 = Bundle By Name(cluster=T6 {"ID"=0, "TimeStamp"=0, "TimeFlag"=0, "SendType"=0, "RemoteFlag"=0, "ExternFlag"=0, "DataLen"=0, "Data"=[], "Reserved"=[]} ("Send"), "ID"=w392, "RemoteFlag"=w404, "ExternFlag"=w403, "DataLen"=u8 3, "Data"=w393) -> (w405:T6)
            n161 = Build Array(w405) -> (w406:T6[])
            n162 = Unbundle By Name(w396) -> ("DevType"=w409:T5, "DevIndex"=w408:u32, "CanIndex"=w407:T4)
            n163 = call "VCI_Transmit.vi"("Buffer"=w406, "CANIndex"=w407, "DevIndex"=w408, "DevType"=w409) -> ()  [unwired: 1 in, 7 out]
          }
          event "速度环KI_W": Value Change {
            w434 = u8 0 items=["数据帧", "遥控帧"]
            w435 = u8 0 items=["标准帧", "扩展帧"]
            # "索引地址"
            n164 = event-data() -> ()  [unwired: 2 out]
            n165 = property on="电机ID" class="CmbBox"() -> ("Value"=w426:string)  [unwired: 2 in, 2 out]
            n166 = Multiply ("乘")(x="速度环KI", y=u16 256) -> (x*y=w439:u16)
            n167 = Scan From String(format string="%x" ("格式字符串"), input string=w426, default 1=u8 0) -> (output 1=w423:u8)  [unwired: 2 in, 3 out]
            n168 = Split Number(x=w439) -> (hi(x)=w440:u8, lo(x)=w441:u8)
            n169 = Add(x=u32 16, y=w423) -> (x+y=w418:u32)
            n170 = Build Array(u8 84, w440, w441) -> (w419:u8[])
            n171 = Bundle By Name(cluster=T6 {"ID"=0, "TimeStamp"=0, "TimeFlag"=0, "SendType"=0, "RemoteFlag"=0, "ExternFlag"=0, "DataLen"=0, "Data"=[], "Reserved"=[]} ("Send"), "ID"=w418, "RemoteFlag"=w434, "ExternFlag"=w435, "DataLen"=u8 3, "Data"=w419) -> (w433:T6)
            n172 = Build Array(w433) -> (w432:T6[])
            n173 = Unbundle By Name(w422) -> ("DevType"=w429:T5, "DevIndex"=w430:u32, "CanIndex"=w431:T4)
            n174 = call "VCI_Transmit.vi"("Buffer"=w432, "CANIndex"=w431, "DevIndex"=w430, "DevType"=w429) -> ()  [unwired: 1 in, 7 out]
          }
          event "加速度_W": Value Change {
            w456 = u8 0 items=["数据帧", "遥控帧"]
            w455 = u8 0 items=["标准帧", "扩展帧"]
            # "索引地址"
            n175 = event-data() -> ()  [unwired: 2 out]
            n176 = property on="电机ID" class="CmbBox"() -> ("Value"=w464:string)  [unwired: 2 in, 2 out]
            n177 = Multiply ("乘")(x="加速度", y=u16 8) -> (x*y=w451:u16)
            n178 = Scan From String(format string="%x" ("格式字符串"), input string=w464, default 1=u8 0) -> (output 1=w467:u8)  [unwired: 2 in, 3 out]
            n179 = Split Number(x=w451) -> (hi(x)=w450:u8, lo(x)=w449:u8)
            n180 = Add(x=u32 16, y=w467) -> (x+y=w444:u32)
            n181 = Build Array(u8 85, w450, w449) -> (w445:u8[])
            n182 = Bundle By Name(cluster=T6 {"ID"=0, "TimeStamp"=0, "TimeFlag"=0, "SendType"=0, "RemoteFlag"=0, "ExternFlag"=0, "DataLen"=0, "Data"=[], "Reserved"=[]} ("Send"), "ID"=w444, "RemoteFlag"=w456, "ExternFlag"=w455, "DataLen"=u8 3, "Data"=w445) -> (w457:T6)
            n183 = Build Array(w457) -> (w458:T6[])
            n184 = Unbundle By Name(w448) -> ("DevType"=w461:T5, "DevIndex"=w460:u32, "CanIndex"=w459:T4)
            n185 = call "VCI_Transmit.vi"("Buffer"=w458, "CANIndex"=w459, "DevIndex"=w460, "DevType"=w461) -> ()  [unwired: 1 in, 7 out]
          }
          event "AI_K0_W": Value Change {
            w480 = u8 0 items=["数据帧", "遥控帧"]
            w479 = u8 0 items=["标准帧", "扩展帧"]
            # "索引地址"
            n186 = event-data() -> ()  [unwired: 2 out]
            n187 = property on="电机ID" class="CmbBox"() -> ("Value"=w488:string)  [unwired: 2 in, 2 out]
            n188 = Scan From String(format string="%x" ("格式字符串"), input string=w488, default 1=u8 0) -> (output 1=w491:u8)  [unwired: 2 in, 3 out]
            n189 = Split Number(x="A电流零偏") -> (hi(x)=w476:u8, lo(x)=w475:u8)
            n190 = Add(x=u32 16, y=w491) -> (x+y=w470:u32)
            n191 = Build Array(u8 90, w476, w475) -> (w471:u8[])
            n192 = Bundle By Name(cluster=T6 {"ID"=0, "TimeStamp"=0, "TimeFlag"=0, "SendType"=0, "RemoteFlag"=0, "ExternFlag"=0, "DataLen"=0, "Data"=[], "Reserved"=[]} ("Send"), "ID"=w470, "RemoteFlag"=w480, "ExternFlag"=w479, "DataLen"=u8 3, "Data"=w471) -> (w481:T6)
            n193 = Build Array(w481) -> (w482:T6[])
            n194 = Unbundle By Name(w474) -> ("DevType"=w485:T5, "DevIndex"=w484:u32, "CanIndex"=w483:T4)
            n195 = call "VCI_Transmit.vi"("Buffer"=w482, "CANIndex"=w483, "DevIndex"=w484, "DevType"=w485) -> ()  [unwired: 1 in, 7 out]
          }
          event "BI_K0_W": Value Change {
            w504 = u8 0 items=["数据帧", "遥控帧"]
            w503 = u8 0 items=["标准帧", "扩展帧"]
            # "索引地址"
            n196 = event-data() -> ()  [unwired: 2 out]
            n197 = property on="电机ID" class="CmbBox"() -> ("Value"=w512:string)  [unwired: 2 in, 2 out]
            n198 = Scan From String(format string="%x" ("格式字符串"), input string=w512, default 1=u8 0) -> (output 1=w515:u8)  [unwired: 2 in, 3 out]
            n199 = Split Number(x="B电流零偏") -> (hi(x)=w500:u8, lo(x)=w499:u8)
            n200 = Add(x=u32 16, y=w515) -> (x+y=w494:u32)
            n201 = Build Array(u8 91, w500, w499) -> (w495:u8[])
            n202 = Bundle By Name(cluster=T6 {"ID"=0, "TimeStamp"=0, "TimeFlag"=0, "SendType"=0, "RemoteFlag"=0, "ExternFlag"=0, "DataLen"=0, "Data"=[], "Reserved"=[]} ("Send"), "ID"=w494, "RemoteFlag"=w504, "ExternFlag"=w503, "DataLen"=u8 3, "Data"=w495) -> (w505:T6)
            n203 = Build Array(w505) -> (w506:T6[])
            n204 = Unbundle By Name(w498) -> ("DevType"=w509:T5, "DevIndex"=w508:u32, "CanIndex"=w507:T4)
            n205 = call "VCI_Transmit.vi"("Buffer"=w506, "CANIndex"=w507, "DevIndex"=w508, "DevType"=w509) -> ()  [unwired: 1 in, 7 out]
          }
          event "CI_K0_W": Value Change {
            w528 = u8 0 items=["数据帧", "遥控帧"]
            w527 = u8 0 items=["标准帧", "扩展帧"]
            # "索引地址"
            n206 = event-data() -> ()  [unwired: 2 out]
            n207 = property on="电机ID" class="CmbBox"() -> ("Value"=w536:string)  [unwired: 2 in, 2 out]
            n208 = Scan From String(format string="%x" ("格式字符串"), input string=w536, default 1=u8 0) -> (output 1=w539:u8)  [unwired: 2 in, 3 out]
            n209 = Split Number(x="C电流零偏") -> (hi(x)=w524:u8, lo(x)=w523:u8)
            n210 = Add(x=u32 16, y=w539) -> (x+y=w518:u32)
            n211 = Build Array(u8 92, w524, w523) -> (w519:u8[])
            n212 = Bundle By Name(cluster=T6 {"ID"=0, "TimeStamp"=0, "TimeFlag"=0, "SendType"=0, "RemoteFlag"=0, "ExternFlag"=0, "DataLen"=0, "Data"=[], "Reserved"=[]} ("Send"), "ID"=w518, "RemoteFlag"=w528, "ExternFlag"=w527, "DataLen"=u8 3, "Data"=w519) -> (w529:T6)
            n213 = Build Array(w529) -> (w530:T6[])
            n214 = Unbundle By Name(w522) -> ("DevType"=w533:T5, "DevIndex"=w532:u32, "CanIndex"=w531:T4)
            n215 = call "VCI_Transmit.vi"("Buffer"=w530, "CANIndex"=w531, "DevIndex"=w532, "DevType"=w533) -> ()  [unwired: 1 in, 7 out]
          }
          event "DATA_SAVE_W": Value Change {
            w558 = u8 0 items=["数据帧", "遥控帧"]
            w559 = u8 0 items=["标准帧", "扩展帧"]
            # "地址"
            n216 = event-data() -> ()  [unwired: 2 out]
            n217 = property on="电机ID" class="CmbBox"() -> ("Value"=w549:string)  [unwired: 2 in, 2 out]
            n218 = Scan From String(format string="%x" ("格式字符串"), input string=w549, default 1=u8 0) -> (output 1=w546:u8)  [unwired: 2 in, 3 out]
            n219 = call "Demo_MakeData.vi"("DataString"="50") -> ("Data"=w543:u8[], "DataLen"=w554:u8)  [unwired: 9 out]
            n220 = Add(x=u32 16, y=w546) -> (x+y=w542:u32)
            n221 = Bundle By Name(cluster=T6 {"ID"=0, "TimeStamp"=0, "TimeFlag"=0, "SendType"=0, "RemoteFlag"=0, "ExternFlag"=0, "DataLen"=0, "Data"=[], "Reserved"=[]} ("Send"), "ID"=w542, "RemoteFlag"=w558, "ExternFlag"=w559, "DataLen"=w554, "Data"=w543) -> (w557:T6)
            n222 = Build Array(w557) -> (w556:T6[])
            n223 = Unbundle By Name(w545) -> ("DevType"=w552:T5, "DevIndex"=w553:u32, "CanIndex"=w555:T4)
            n224 = call "VCI_Transmit.vi"("Buffer"=w556, "CANIndex"=w555, "DevIndex"=w553, "DevType"=w552) -> ()  [unwired: 1 in, 7 out]
          }
          event "设定位置_R": Value Change {
            w569 = u8 0 items=["数据帧", "遥控帧"]
            w568 = u8 0 items=["标准帧", "扩展帧"]
            # "地址"
            n225 = event-data() -> ()  [unwired: 2 out]
            n226 = property on="电机ID" class="CmbBox"() -> ("Value"=w578:string)  [unwired: 2 in, 2 out]
            n227 = Scan From String(format string="%x" ("格式字符串"), input string=w578, default 1=u8 0) -> (output 1=w581:u8)  [unwired: 2 in, 3 out]
            n228 = call "Demo_MakeData.vi"("DataString"="40 ") -> ("Data"=w564:u8[], "DataLen"=w573:u8)  [unwired: 9 out]
            n229 = Add(x=u32 48, y=w581) -> (x+y=w563:u32)
            n230 = Bundle By Name(cluster=T6 {"ID"=0, "TimeStamp"=0, "TimeFlag"=0, "SendType"=0, "RemoteFlag"=0, "ExternFlag"=0, "DataLen"=0, "Data"=[], "Reserved"=[]} ("Send"), "ID"=w563, "RemoteFlag"=w569, "ExternFlag"=w568, "DataLen"=w573, "Data"=w564) -> (w570:T6)
            n231 = Build Array(w570) -> (w571:T6[])
            n232 = Unbundle By Name(w566) -> ("DevType"=w575:T5, "DevIndex"=w574:u32, "CanIndex"=w572:T4)
            n233 = call "VCI_Transmit.vi"("Buffer"=w571, "CANIndex"=w572, "DevIndex"=w574, "DevType"=w575) -> ()  [unwired: 1 in, 7 out]
          }
          event "设定速度_R": Value Change {
            w600 = u8 0 items=["数据帧", "遥控帧"]
            w601 = u8 0 items=["标准帧", "扩展帧"]
            # "地址"
            n234 = event-data() -> ()  [unwired: 2 out]
            n235 = property on="电机ID" class="CmbBox"() -> ("Value"=w591:string)  [unwired: 2 in, 2 out]
            n236 = Scan From String(format string="%x" ("格式字符串"), input string=w591, default 1=u8 0) -> (output 1=w588:u8)  [unwired: 2 in, 3 out]
            n237 = call "Demo_MakeData.vi"("DataString"="41 ") -> ("Data"=w585:u8[], "DataLen"=w596:u8)  [unwired: 9 out]
            n238 = Add(x=u32 48, y=w588) -> (x+y=w584:u32)
            n239 = Bundle By Name(cluster=T6 {"ID"=0, "TimeStamp"=0, "TimeFlag"=0, "SendType"=0, "RemoteFlag"=0, "ExternFlag"=0, "DataLen"=0, "Data"=[], "Reserved"=[]} ("Send"), "ID"=w584, "RemoteFlag"=w600, "ExternFlag"=w601, "DataLen"=w596, "Data"=w585) -> (w599:T6)
            n240 = Build Array(w599) -> (w598:T6[])
            n241 = Unbundle By Name(w587) -> ("DevType"=w594:T5, "DevIndex"=w595:u32, "CanIndex"=w597:T4)
            n242 = call "VCI_Transmit.vi"("Buffer"=w598, "CANIndex"=w597, "DevIndex"=w595, "DevType"=w594) -> ()  [unwired: 1 in, 7 out]
          }
          event "设定电流_R": Value Change {
            w621 = u8 0 items=["数据帧", "遥控帧"]
            w622 = u8 0 items=["标准帧", "扩展帧"]
            # "地址"
            n243 = event-data() -> ()  [unwired: 2 out]
            n244 = property on="电机ID" class="CmbBox"() -> ("Value"=w612:string)  [unwired: 2 in, 2 out]
            n245 = Scan From String(format string="%x" ("格式字符串"), input string=w612, default 1=u8 0) -> (output 1=w609:u8)  [unwired: 2 in, 3 out]
            n246 = call "Demo_MakeData.vi"("DataString"="42 ") -> ("Data"=w606:u8[], "DataLen"=w617:u8)  [unwired: 9 out]
            n247 = Add(x=u32 48, y=w609) -> (x+y=w605:u32)
            n248 = Bundle By Name(cluster=T6 {"ID"=0, "TimeStamp"=0, "TimeFlag"=0, "SendType"=0, "RemoteFlag"=0, "ExternFlag"=0, "DataLen"=0, "Data"=[], "Reserved"=[]} ("Send"), "ID"=w605, "RemoteFlag"=w621, "ExternFlag"=w622, "DataLen"=w617, "Data"=w606) -> (w620:T6)
            n249 = Build Array(w620) -> (w619:T6[])
            n250 = Unbundle By Name(w608) -> ("DevType"=w615:T5, "DevIndex"=w616:u32, "CanIndex"=w618:T4)
            n251 = call "VCI_Transmit.vi"("Buffer"=w619, "CANIndex"=w618, "DevIndex"=w616, "DevType"=w615) -> ()  [unwired: 1 in, 7 out]
          }
          event "电流环KP_R": Value Change {
            w642 = u8 0 items=["数据帧", "遥控帧"]
            w643 = u8 0 items=["标准帧", "扩展帧"]
            # "地址"
            n252 = event-data() -> ()  [unwired: 2 out]
            n253 = property on="电机ID" class="CmbBox"() -> ("Value"=w633:string)  [unwired: 2 in, 2 out]
            n254 = Scan From String(format string="%x" ("格式字符串"), input string=w633, default 1=u8 0) -> (output 1=w630:u8)  [unwired: 2 in, 3 out]
            n255 = call "Demo_MakeData.vi"("DataString"="51 ") -> ("Data"=w627:u8[], "DataLen"=w638:u8)  [unwired: 9 out]
            n256 = Add(x=u32 48, y=w630) -> (x+y=w626:u32)
            n257 = Bundle By Name(cluster=T6 {"ID"=0, "TimeStamp"=0, "TimeFlag"=0, "SendType"=0, "RemoteFlag"=0, "ExternFlag"=0, "DataLen"=0, "Data"=[], "Reserved"=[]} ("Send"), "ID"=w626, "RemoteFlag"=w642, "ExternFlag"=w643, "DataLen"=w638, "Data"=w627) -> (w641:T6)
            n258 = Build Array(w641) -> (w640:T6[])
            n259 = Unbundle By Name(w629) -> ("DevType"=w636:T5, "DevIndex"=w637:u32, "CanIndex"=w639:T4)
            n260 = call "VCI_Transmit.vi"("Buffer"=w640, "CANIndex"=w639, "DevIndex"=w637, "DevType"=w636) -> ()  [unwired: 1 in, 7 out]
          }
          event "电流环KI_R": Value Change {
            w663 = u8 0 items=["数据帧", "遥控帧"]
            w664 = u8 0 items=["标准帧", "扩展帧"]
            # "地址"
            n261 = event-data() -> ()  [unwired: 2 out]
            n262 = property on="电机ID" class="CmbBox"() -> ("Value"=w654:string)  [unwired: 2 in, 2 out]
            n263 = Scan From String(format string="%x" ("格式字符串"), input string=w654, default 1=u8 0) -> (output 1=w651:u8)  [unwired: 2 in, 3 out]
            n264 = call "Demo_MakeData.vi"("DataString"="52 ") -> ("Data"=w648:u8[], "DataLen"=w659:u8)  [unwired: 9 out]
            n265 = Add(x=u32 48, y=w651) -> (x+y=w647:u32)
            n266 = Bundle By Name(cluster=T6 {"ID"=0, "TimeStamp"=0, "TimeFlag"=0, "SendType"=0, "RemoteFlag"=0, "ExternFlag"=0, "DataLen"=0, "Data"=[], "Reserved"=[]} ("Send"), "ID"=w647, "RemoteFlag"=w663, "ExternFlag"=w664, "DataLen"=w659, "Data"=w648) -> (w662:T6)
            n267 = Build Array(w662) -> (w661:T6[])
            n268 = Unbundle By Name(w650) -> ("DevType"=w657:T5, "DevIndex"=w658:u32, "CanIndex"=w660:T4)
            n269 = call "VCI_Transmit.vi"("Buffer"=w661, "CANIndex"=w660, "DevIndex"=w658, "DevType"=w657) -> ()  [unwired: 1 in, 7 out]
          }
          event "速度环KP_R": Value Change {
            w674 = u8 0 items=["数据帧", "遥控帧"]
            w673 = u8 0 items=["标准帧", "扩展帧"]
            # "地址"
            n270 = event-data() -> ()  [unwired: 2 out]
            n271 = property on="电机ID" class="CmbBox"() -> ("Value"=w683:string)  [unwired: 2 in, 2 out]
            n272 = Scan From String(format string="%x" ("格式字符串"), input string=w683, default 1=u8 0) -> (output 1=w686:u8)  [unwired: 2 in, 3 out]
            n273 = call "Demo_MakeData.vi"("DataString"="53 ") -> ("Data"=w669:u8[], "DataLen"=w678:u8)  [unwired: 9 out]
            n274 = Add(x=u32 48, y=w686) -> (x+y=w668:u32)
            n275 = Bundle By Name(cluster=T6 {"ID"=0, "TimeStamp"=0, "TimeFlag"=0, "SendType"=0, "RemoteFlag"=0, "ExternFlag"=0, "DataLen"=0, "Data"=[], "Reserved"=[]} ("Send"), "ID"=w668, "RemoteFlag"=w674, "ExternFlag"=w673, "DataLen"=w678, "Data"=w669) -> (w675:T6)
            n276 = Build Array(w675) -> (w676:T6[])
            n277 = Unbundle By Name(w671) -> ("DevType"=w680:T5, "DevIndex"=w679:u32, "CanIndex"=w677:T4)
            n278 = call "VCI_Transmit.vi"("Buffer"=w676, "CANIndex"=w677, "DevIndex"=w679, "DevType"=w680) -> ()  [unwired: 1 in, 7 out]
          }
          event "速度环KI_R": Value Change {
            w695 = u8 0 items=["数据帧", "遥控帧"]
            w694 = u8 0 items=["标准帧", "扩展帧"]
            # "地址"
            n279 = event-data() -> ()  [unwired: 2 out]
            n280 = property on="电机ID" class="CmbBox"() -> ("Value"=w704:string)  [unwired: 2 in, 2 out]
            n281 = Scan From String(format string="%x" ("格式字符串"), input string=w704, default 1=u8 0) -> (output 1=w707:u8)  [unwired: 2 in, 3 out]
            n282 = call "Demo_MakeData.vi"("DataString"="54 ") -> ("Data"=w690:u8[], "DataLen"=w699:u8)  [unwired: 9 out]
            n283 = Add(x=u32 48, y=w707) -> (x+y=w689:u32)
            n284 = Bundle By Name(cluster=T6 {"ID"=0, "TimeStamp"=0, "TimeFlag"=0, "SendType"=0, "RemoteFlag"=0, "ExternFlag"=0, "DataLen"=0, "Data"=[], "Reserved"=[]} ("Send"), "ID"=w689, "RemoteFlag"=w695, "ExternFlag"=w694, "DataLen"=w699, "Data"=w690) -> (w696:T6)
            n285 = Build Array(w696) -> (w697:T6[])
            n286 = Unbundle By Name(w692) -> ("DevType"=w701:T5, "DevIndex"=w700:u32, "CanIndex"=w698:T4)
            n287 = call "VCI_Transmit.vi"("Buffer"=w697, "CANIndex"=w698, "DevIndex"=w700, "DevType"=w701) -> ()  [unwired: 1 in, 7 out]
          }
          event "加速度_R": Value Change {
            w726 = u8 0 items=["数据帧", "遥控帧"]
            w727 = u8 0 items=["标准帧", "扩展帧"]
            # "地址"
            n288 = event-data() -> ()  [unwired: 2 out]
            n289 = property on="电机ID" class="CmbBox"() -> ("Value"=w717:string)  [unwired: 2 in, 2 out]
            n290 = Scan From String(format string="%x" ("格式字符串"), input string=w717, default 1=u8 0) -> (output 1=w714:u8)  [unwired: 2 in, 3 out]
            n291 = call "Demo_MakeData.vi"("DataString"="55") -> ("Data"=w711:u8[], "DataLen"=w722:u8)  [unwired: 9 out]
            n292 = Add(x=u32 48, y=w714) -> (x+y=w710:u32)
            n293 = Bundle By Name(cluster=T6 {"ID"=0, "TimeStamp"=0, "TimeFlag"=0, "SendType"=0, "RemoteFlag"=0, "ExternFlag"=0, "DataLen"=0, "Data"=[], "Reserved"=[]} ("Send"), "ID"=w710, "RemoteFlag"=w726, "ExternFlag"=w727, "DataLen"=w722, "Data"=w711) -> (w725:T6)
            n294 = Build Array(w725) -> (w724:T6[])
            n295 = Unbundle By Name(w713) -> ("DevType"=w720:T5, "DevIndex"=w721:u32, "CanIndex"=w723:T4)
            n296 = call "VCI_Transmit.vi"("Buffer"=w724, "CANIndex"=w723, "DevIndex"=w721, "DevType"=w720) -> ()  [unwired: 1 in, 7 out]
          }
          event "AI_K0_R": Value Change {
            w737 = u8 0 items=["数据帧", "遥控帧"]
            w736 = u8 0 items=["标准帧", "扩展帧"]
            # "地址"
            n297 = event-data() -> ()  [unwired: 2 out]
            n298 = property on="电机ID" class="CmbBox"() -> ("Value"=w746:string)  [unwired: 2 in, 2 out]
            n299 = Scan From String(format string="%x" ("格式字符串"), input string=w746, default 1=u8 0) -> (output 1=w749:u8)  [unwired: 2 in, 3 out]
            n300 = call "Demo_MakeData.vi"("DataString"="5A") -> ("Data"=w732:u8[], "DataLen"=w741:u8)  [unwired: 9 out]
            n301 = Add(x=u32 48, y=w749) -> (x+y=w731:u32)
            n302 = Bundle By Name(cluster=T6 {"ID"=0, "TimeStamp"=0, "TimeFlag"=0, "SendType"=0, "RemoteFlag"=0, "ExternFlag"=0, "DataLen"=0, "Data"=[], "Reserved"=[]} ("Send"), "ID"=w731, "RemoteFlag"=w737, "ExternFlag"=w736, "DataLen"=w741, "Data"=w732) -> (w738:T6)
            n303 = Build Array(w738) -> (w739:T6[])
            n304 = Unbundle By Name(w734) -> ("DevType"=w743:T5, "DevIndex"=w742:u32, "CanIndex"=w740:T4)
            n305 = call "VCI_Transmit.vi"("Buffer"=w739, "CANIndex"=w740, "DevIndex"=w742, "DevType"=w743) -> ()  [unwired: 1 in, 7 out]
          }
          event "BI_K0_R": Value Change {
            w758 = u8 0 items=["数据帧", "遥控帧"]
            w757 = u8 0 items=["标准帧", "扩展帧"]
            # "地址"
            n306 = event-data() -> ()  [unwired: 2 out]
            n307 = property on="电机ID" class="CmbBox"() -> ("Value"=w767:string)  [unwired: 2 in, 2 out]
            n308 = Scan From String(format string="%x" ("格式字符串"), input string=w767, default 1=u8 0) -> (output 1=w770:u8)  [unwired: 2 in, 3 out]
            n309 = call "Demo_MakeData.vi"("DataString"="5B") -> ("Data"=w753:u8[], "DataLen"=w762:u8)  [unwired: 9 out]
            n310 = Add(x=u32 48, y=w770) -> (x+y=w752:u32)
            n311 = Bundle By Name(cluster=T6 {"ID"=0, "TimeStamp"=0, "TimeFlag"=0, "SendType"=0, "RemoteFlag"=0, "ExternFlag"=0, "DataLen"=0, "Data"=[], "Reserved"=[]} ("Send"), "ID"=w752, "RemoteFlag"=w758, "ExternFlag"=w757, "DataLen"=w762, "Data"=w753) -> (w759:T6)
            n312 = Build Array(w759) -> (w760:T6[])
            n313 = Unbundle By Name(w755) -> ("DevType"=w764:T5, "DevIndex"=w763:u32, "CanIndex"=w761:T4)
            n314 = call "VCI_Transmit.vi"("Buffer"=w760, "CANIndex"=w761, "DevIndex"=w763, "DevType"=w764) -> ()  [unwired: 1 in, 7 out]
          }
          event "CI_K0_R": Value Change {
            w779 = u8 0 items=["数据帧", "遥控帧"]
            w778 = u8 0 items=["标准帧", "扩展帧"]
            # "地址"
            n315 = event-data() -> ()  [unwired: 2 out]
            n316 = property on="电机ID" class="CmbBox"() -> ("Value"=w788:string)  [unwired: 2 in, 2 out]
            n317 = Scan From String(format string="%x" ("格式字符串"), input string=w788, default 1=u8 0) -> (output 1=w791:u8)  [unwired: 2 in, 3 out]
            n318 = call "Demo_MakeData.vi"("DataString"="5C") -> ("Data"=w774:u8[], "DataLen"=w783:u8)  [unwired: 9 out]
            n319 = Add(x=u32 48, y=w791) -> (x+y=w773:u32)
            n320 = Bundle By Name(cluster=T6 {"ID"=0, "TimeStamp"=0, "TimeFlag"=0, "SendType"=0, "RemoteFlag"=0, "ExternFlag"=0, "DataLen"=0, "Data"=[], "Reserved"=[]} ("Send"), "ID"=w773, "RemoteFlag"=w779, "ExternFlag"=w778, "DataLen"=w783, "Data"=w774) -> (w780:T6)
            n321 = Build Array(w780) -> (w781:T6[])
            n322 = Unbundle By Name(w776) -> ("DevType"=w785:T5, "DevIndex"=w784:u32, "CanIndex"=w782:T4)
            n323 = call "VCI_Transmit.vi"("Buffer"=w781, "CANIndex"=w782, "DevIndex"=w784, "DevType"=w785) -> ()  [unwired: 1 in, 7 out]
          }
          event "保存": Value Change {
            w817 = "-"
            n324 = event-data() -> ()  [unwired: 2 out]
            n325 = Get Date/Time String(want seconds? (F)=TRUE) -> (date string=w797:string, time string=w818:string)  [unwired: 2 in]
            n326 = Search and Replace String(input string=w797, search string="/", replace string="-") -> (result string=w803:string)  [unwired: 5 in, 3 out]
            n327 = Search and Replace String(input string=w818, search string=":", replace string="-") -> (result string=w815:string)  [unwired: 5 in, 3 out]
            n328 = property on="保存_S" class="Bool (严格)"() -> ("Value"=w809:bool)  [unwired: 2 in, 2 out]
            n329 = Search and Replace String(input string=w803, search string="/", replace string="-") -> (result string=w798:string)  [unwired: 5 in, 3 out]
            n330 = Search and Replace String(input string=w815, search string=":", replace string="-") -> (result string=w816:string)  [unwired: 5 in, 3 out]
            n331 = Not(x=w809) -> (.not. x?=w805:bool)
            n332 = property on="保存_S" class="Bool (严格)"("Value"=w805) -> ()  [unwired: 2 in, 2 out]
            n333 = Concatenate Strings("D:\\PMSM\\", w798, w817, w816, w817, "电机数据存储", ".txt") -> (w795:string)
            n334 = Select(t=w795, s=w805, f="") -> (s? t:f=w810:string)
            n335 = String To Path(string=w810) -> (path=w796:path)
            n336 = local write "存储路径"(w796) -> ()
          }
          event "Close": Value Change {
            w830 = T10 1 items=["OK"=1, "ERROR1"=0, "ERROR2"=-1] ("y")
            n337 = event-data() -> ()  [unwired: 2 out]
            n338 = Unbundle By Name(w834) -> ("DevType"=w833:T5, "DevIndex"=w832:u32)
            n339 = call "VCI_CloseDevice.vi"("DevIndex"=w832, "DevType"=w833) -> ("Return Val"=w831:T10)  [unwired: 1 in, 8 out]
            n340 = Equal?(x=w831, y=w830) -> (x = y?=w828:bool)
            n341 = Not(x=w828) -> (.not. x?=w824:bool)
            n342 = Bundle By Name(cluster=cluster{"CANOpen":bool} {"CANOpen"=FALSE} ("事件数据"), "CANOpen"=w824) -> (w823:cluster{"CANOpen":bool})
            n343 = Bundle By Name(cluster=w829, "Open"=w824) -> (w827:cluster{"Open":bool, "SendCnt":u32})
            n344 = local write "Open"(w824) -> ()
            n345 = Generate User Event(user event=w826, event data cluster=w823) -> ()  [unwired: 1 in, 2 out]
          }
          event User Event {
            w844 = u8 0
            w843 = u8 2
            n346 = event-data() -> ("CANOpen"=w837:bool)  [unwired: 1 out]
            "Open" <- w837
            n347 = Not(x=w837) -> (.not. x?=w838:bool)
            n348 = Select(t=w843, s=w837, f=w844) -> (s? t:f=w845:u8)
            n349 = Select(t=w844, s=w837, f=w843) -> (s? t:f=w836:u8)
            n350 = property class="VI"("Front Panel.Closeable"=w838) -> ()  [unwired: 2 in, 2 out]
            n351 = property on="Close" class="Bool"("DisabledEnum"=w836) -> ()  [unwired: 2 in, 2 out]
            n352 = property on="ID" class="DigNum (严格)"("DisabledEnum"=w836) -> ()  [unwired: 2 in, 2 out]
            n353 = property on="Data" class="Str"("DisabledEnum"=w836) -> ()  [unwired: 2 in, 2 out]
            n354 = property on="Format" class="Ring (严格)"("DisabledEnum"=w836) -> ()  [unwired: 2 in, 2 out]
            n355 = property on="Type" class="Ring (严格)"("DisabledEnum"=w836) -> ()  [unwired: 2 in, 2 out]
            n356 = property on="Send" class="Bool"("DisabledEnum"=w836) -> ()  [unwired: 2 in, 2 out]
            n357 = Select(t=enum16{"Init", "Wait", "Run", "Exit"}."Run", s=w837, f=enum16{"Init", "Wait", "Run", "Exit"}."Wait") -> (s? t:f=w840:enum16{"Init", "Wait", "Run", "Exit"})
            n358 = property on="Fliter" class="Ring (严格)"("DisabledEnum"=w845) -> ()  [unwired: 2 in, 2 out]
            n359 = property on="DevType" class="Ring (严格)"("DisabledEnum"=w845) -> ()  [unwired: 2 in, 2 out]
            n360 = property on="Channel" class="Ring (严格)"("DisabledEnum"=w845) -> ()  [unwired: 2 in, 2 out]
            n361 = property on="AccCode" class="DigNum (严格)"("DisabledEnum"=w845) -> ()  [unwired: 2 in, 2 out]
            n362 = property on="AccMask" class="DigNum (严格)"("DisabledEnum"=w845) -> ()  [unwired: 2 in, 2 out]
            n363 = property on="InitFlag" class="Ring (严格)"("DisabledEnum"=w845) -> ()  [unwired: 2 in, 2 out]
            n364 = property on="Mode" class="Ring (严格)"("DisabledEnum"=w845) -> ()  [unwired: 2 in, 2 out]
            n365 = property on="kBaudRate" class="Ring (严格)"("DisabledEnum"=w845) -> ()  [unwired: 2 in, 2 out]
            n366 = property on="电机ID_W" class="Bool"("DisabledEnum"=w836) -> ()  [unwired: 2 in, 2 out]
            n367 = property on="监测_W" class="Bool"("DisabledEnum"=w836) -> ()  [unwired: 2 in, 2 out]
            n368 = property on="模式_W" class="Bool"("DisabledEnum"=w836) -> ()  [unwired: 2 in, 2 out]
            n369 = property on="模式_R" class="Bool"("DisabledEnum"=w836) -> ()  [unwired: 2 in, 2 out]
            n370 = property on="设定位置_W" class="Bool"("DisabledEnum"=w836) -> ()  [unwired: 2 in, 2 out]
            n371 = property on="设定位置_R" class="Bool"("DisabledEnum"=w836) -> ()  [unwired: 2 in, 2 out]
            n372 = property on="设定速度_W" class="Bool"("DisabledEnum"=w836) -> ()  [unwired: 2 in, 2 out]
            n373 = property on="设定速度_R" class="Bool"("DisabledEnum"=w836) -> ()  [unwired: 2 in, 2 out]
            n374 = property on="设定电流_W" class="Bool"("DisabledEnum"=w836) -> ()  [unwired: 2 in, 2 out]
            n375 = property on="设定电流_R" class="Bool"("DisabledEnum"=w836) -> ()  [unwired: 2 in, 2 out]
            n376 = property on="保存" class="Bool"("DisabledEnum"=w836) -> ()  [unwired: 2 in, 2 out]
            n377 = property on="电流环KP_W" class="Bool"("DisabledEnum"=w836) -> ()  [unwired: 2 in, 2 out]
            n378 = property on="电流环KI_W" class="Bool"("DisabledEnum"=w836) -> ()  [unwired: 2 in, 2 out]
            n379 = property on="速度环KP_W" class="Bool"("DisabledEnum"=w836) -> ()  [unwired: 2 in, 2 out]
            n380 = property on="速度环KI_W" class="Bool"("DisabledEnum"=w836) -> ()  [unwired: 2 in, 2 out]
            n381 = property on="加速度_W" class="Bool"("DisabledEnum"=w836) -> ()  [unwired: 2 in, 2 out]
            n382 = property on="AI_K0_W" class="Bool"("DisabledEnum"=w836) -> ()  [unwired: 2 in, 2 out]
            n383 = property on="BI_K0_W" class="Bool"("DisabledEnum"=w836) -> ()  [unwired: 2 in, 2 out]
            n384 = property on="CI_K0_W" class="Bool"("DisabledEnum"=w836) -> ()  [unwired: 2 in, 2 out]
            n385 = property on="DATA_SAVE_W" class="Bool"("DisabledEnum"=w836) -> ()  [unwired: 2 in, 2 out]
            n386 = property on="电流环KP_R" class="Bool"("DisabledEnum"=w836) -> ()  [unwired: 2 in, 2 out]
            n387 = property on="电流环KI_R" class="Bool"("DisabledEnum"=w836) -> ()  [unwired: 2 in, 2 out]
            n388 = property on="速度环KP_R" class="Bool"("DisabledEnum"=w836) -> ()  [unwired: 2 in, 2 out]
            n389 = property on="速度环KI_R" class="Bool"("DisabledEnum"=w836) -> ()  [unwired: 2 in, 2 out]
            n390 = property on="加速度_R" class="Bool"("DisabledEnum"=w836) -> ()  [unwired: 2 in, 2 out]
            n391 = property on="AI_K0_R" class="Bool"("DisabledEnum"=w836) -> ()  [unwired: 2 in, 2 out]
            n392 = property on="BI_K0_R" class="Bool"("DisabledEnum"=w836) -> ()  [unwired: 2 in, 2 out]
            n393 = property on="CI_K0_R" class="Bool"("DisabledEnum"=w836) -> ()  [unwired: 2 in, 2 out]
          }
        }
        "数组" <- w150
        "CAN ID" <- w149
      }
      frame "Exit" {
        n394 = Release Queue(queue=w856) -> ()  [unwired: 1 in, 4 out]
        n395 = Unregister For Events(event registration refnum=w855) -> (error out=w854:errorcluster)  [unwired: 1 in]
        n396 = Destroy User Event(user event=w853, error in=w854) -> ()  [unwired: 1 out]
        n397 = Unbundle By Name(w852) -> ("Open"=w851:bool)
        n398 = case shown="真" w851 {
          tunnel: w850 -> [_ w860]
          frame False {
          }
          frame True {
            n399 = Unbundle By Name(w860) -> ("DevType"=w859:T5, "DevIndex"=w858:u32)
            n400 = call "VCI_CloseDevice.vi"("DevIndex"=w858, "DevType"=w859) -> ()  [unwired: 1 in, 9 out]
          }
        }
        n401 = local write "RcvEnable"(FALSE ("RcvEnable")) -> ()
      }
    }
  }
  n402 = while "数据更新线程" {
    tunnel: w9 -> [w866]
    shift-right: [w861] -> _
    shift-left: u32 0 ("RecvCnt") -> [w862]
    stop <- w865 stop-if-true
    n403 = Dequeue Element(queue=w866) -> (element=w864:T7, timed out?=w863:bool, error out=w865:errorcluster)  [unwired: 2 in, 1 out]
    n404 = case shown="假" w863 {
      tunnel: w864 -> [w876 _]
      tunnel: w862 -> [w870 w1220]
      tunnel: [w869 w1220] -> w861
      frame False {
        n405 = Array To Cluster(array=w876) -> (cluster=w878:T12)
        n406 = Unbundle By Name(w878) -> ("[0]"=w877:T13)
        n407 = Increment(x=w870) -> (x+1=w869:u32)
        "sCnt" <- w869
        n408 = Unbundle By Name(w877) -> ("VCI_CAN_OBJ"=w875:T6)  [unwired: 3 out]
        n409 = Unbundle By Name(w875) -> ("ID"=w873:u32, "Data"=w874:u8[])  [unwired: 7 out]
        "CAN STD_ID" <- w873
        n410 = And(x=w873, y=u32 15) -> (x .and. y?=→"电机ID_R":u32)
        n411 = And(x=w873, y=u32 240) -> (x .and. y?=w868:u32)
        n412 = case shown="40" w868 {
          tunnel: w874 -> [_ w884]
          frame 0, Default {
          }
          frame 64 {
            n413 = local read "存储路径"() -> (w880:path)
            n414 = local read "保存_S"() -> (w881:bool)
            n415 = Index Array(array=w884, index=0) -> (element=w883:u8)
            n416 = case shown="31" w883 {
              tunnel: w884 -> [_ w912 w925 w936 w955 w975 w999 w1016 w1036 w1049 w1074 w1093 w1096 w1103 w1111 w1121 w1127 w1140 w1143 w1153 w1163 w1173 w1183 w1193 w1206 w1209 w1215]
              tunnel: [_ _ _ _ w943 w965 w988 w1014 w1031 w1048 w1063 w1087 _ _ _ _ _ _ _ _ _ _ _ _ _ _ _] -> w879
              frame 0, Default {
              }
              frame 32 {
                n417 = Array To Cluster(array=w912) -> (cluster=w913:T14)
                n418 = Unbundle By Name(w913) -> ("Data[1]"=w911:u8)  [unwired: 1 out]
                n419 = To Unsigned Byte Integer(number=w911) -> (unsigned 8bit integer=w908:u8)
                n420 = Number To Hexadecimal String(1:2, 2:w908) -> (0:w909:string)
                n421 = property on="模式_回" class="CmbBox"("Value"=w909) -> ()  [unwired: 2 in, 2 out]
              }
              frame 33 {
                n422 = Array To Cluster(array=w925) -> (cluster=w927:T14)
                n423 = Unbundle By Name(w927) -> ("Data[1]"=w926:u8)  [unwired: 1 out]
                n424 = To Unsigned Byte Integer(number=w926) -> (unsigned 8bit integer=w924:u8)
                n425 = Number To Boolean Array(number=w924) -> (Boolean array=w923:bool[])
                n426 = Array To Cluster(array=w923) -> (cluster=w922:T15)
                n427 = Unbundle(w922) -> ("Boolean array[0]"=→"warn0":bool, "Boolean array[1]"=→"warn1":bool, "Boolean array[2]"=→"高温":bool, "Boolean array[3]"=→"warn3":bool, "Boolean array[4]"=→"warn4":bool, "Boolean array[5]"=→"warn5":bool, "Boolean array[6]"=→"warn6":bool, "Boolean array[7]"=→"warn7":bool)
              }
              frame 34 {
                n428 = Array To Cluster(array=w936) -> (cluster=w941:T14)
                n429 = Unbundle By Name(w941) -> ("Data[1]"=w940:u8)  [unwired: 1 out]
                n430 = To Unsigned Byte Integer(number=w940) -> (unsigned 8bit integer=w939:u8)
                n431 = Number To Boolean Array(number=w939) -> (Boolean array=w938:bool[])
                n432 = Array To Cluster(array=w938) -> (cluster=w937:T15)
                n433 = Unbundle(w937) -> ("Boolean array[0]"=→"低压":bool, "Boolean array[1]"=→"高压":bool, "Boolean array[2]"=→"高温":bool, "Boolean array[3]"=→"ERRO3":bool, "Boolean array[4]"=→"ERRO4":bool, "Boolean array[5]"=→"ERRO5":bool, "Boolean array[6]"=→"ERRO6":bool, "Boolean array[7]"=→"ERRO7":bool)
              }
              frame 49 {
                w944 = 0.0054931640625
                w957 = 8
                n434 = Array To Cluster(array=w955) -> (cluster=w961:T14)
                n435 = Unbundle By Name(w961) -> ("Data[1]"=w949:u8, "Data[2]"=w950:u8, "Data[3]"=w951:u8, "Data[4]"=w952:u8, "Data[5]"=w948:u8, "Data[6]"=w947:u8)  [unwired: 1 out]
                n436 = Join Numbers(hi=w948, lo=w947) -> ((hi.lo)=w946:u16)
                n437 = To Unsigned Word Integer(number=w949) -> (unsigned 16bit integer=w964:u16)
                n438 = To Unsigned Word Integer(number=w951) -> (unsigned 16bit integer=w960:u16)
                n439 = To Word Integer(number=w946) -> (16bit integer=w945:i16)
                n440 = Rotate(1:w964, 2:w957) -> (0:w963:u16)
                n441 = Rotate(1:w960, 2:w957) -> (0:w959:u16)
                n442 = Add(x=w963, y=w950) -> (x+y=w962:u16)
                n443 = Add(x=w959, y=w952) -> (x+y=w958:u16)
                n444 = Multiply(x=w962, y=w944) -> (x*y=w954:dbl)
                "机械角度" <- w954
                n445 = Multiply(x=w958, y=w944) -> (x*y=w953:dbl)
                "电气角度" <- w953
                n446 = Divide(x=w945, y=1.0) -> (x/y=w942:dbl)
                "转速" <- w942
                "转速" <- w942
                n447 = Build Array(w954, w953, w942) -> (w943:dbl[])
              }
              frame 50 {
                w976 = i16 1024
                w977 = 8
                n448 = Array To Cluster(array=w975) -> (cluster=w984:T14)
                n449 = Unbundle By Name(w984) -> ("Data[1]"=w974:u8, "Data[2]"=w973:u8, "Data[3]"=w972:u8, "Data[4]"=w971:u8, "Data[5]"=w970:u8, "Data[6]"=w969:u8)  [unwired: 1 out]
                n450 = To Word Integer(number=w974) -> (16bit integer=w987:i16)
                n451 = To Word Integer(number=w970) -> (16bit integer=w980:i16)
                n452 = To Word Integer(number=w972) -> (16bit integer=w983:i16)
                n453 = Rotate(1:w987, 2:w977) -> (0:w986:i16)
                n454 = Rotate(1:w980, 2:w977) -> (0:w979:i16)
                n455 = Rotate(1:w983, 2:w977) -> (0:w982:i16)
                n456 = Add(x=w986, y=w973) -> (x+y=w985:i16)
                n457 = Add(x=w979, y=w969) -> (x+y=w978:i16)
                n458 = Add(x=w982, y=w971) -> (x+y=w981:i16)
                n459 = Divide(x=w985, y=w976) -> (x/y=w968:dbl)
                "A电流" <- w968
                "波形图表1" <- w968
                n460 = Divide(x=w978, y=w976) -> (x/y=w966:dbl)
                "C电流" <- w966
                "波形图表3" <- w966
                n461 = Divide(x=w981, y=w976) -> (x/y=w967:dbl)
                "B电流" <- w967
                "波形图表2" <- w967
                n462 = Build Array(w968, w967, w966) -> (w965:dbl[])
              }
              frame 51 {
                w1001 = i16 256
                w1000 = 8
                n463 = Array To Cluster(array=w999) -> (cluster=w1008:T14)
                n464 = Unbundle By Name(w1008) -> ("Data[1]"=w998:u8, "Data[2]"=w997:u8, "Data[3]"=w996:u8, "Data[4]"=w995:u8, "Data[5]"=w994:u8, "Data[6]"=w993:u8)  [unwired: 1 out]
                n465 = To Unsigned Word Integer(number=w998) -> (unsigned 16bit integer=w1011:u16)
                n466 = To Word Integer(number=w996) -> (16bit integer=w1007:i16)
                n467 = To Word Integer(number=w994) -> (16bit integer=w1004:i16)
                n468 = Rotate(1:w1011, 2:w1000) -> (0:w1010:u16)
                n469 = Rotate(1:w1007, 2:w1000) -> (0:w1006:i16)
                n470 = Rotate(1:w1004, 2:w1000) -> (0:w1003:i16)
                n471 = Add(x=w1010, y=w997) -> (x+y=w1009:u16)
                n472 = Add(x=w1006, y=w995) -> (x+y=w1005:i16)
                n473 = Add(x=w1003, y=w993) -> (x+y=w1002:i16)
                n474 = Divide(x=w1009, y=i16 1024) -> (x/y=w991:dbl)
                "供电电压" <- w991
                n475 = Divide(x=w1005, y=w1001) -> (x/y=w990:dbl)
                "Ialfa" <- w990
                n476 = Divide(x=w1002, y=w1001) -> (x/y=w989:dbl)
                "Ibeta" <- w989
                n477 = Build Array(w991, w990, w989) -> (w988:dbl[])
              }
              frame 52 {
                w1015 = i16 256
                w1021 = 8
                n478 = Array To Cluster(array=w1016) -> (cluster=w1025:T14)
                n479 = Unbundle By Name(w1025) -> ("Data[1]"=w1020:u8, "Data[2]"=w1019:u8, "Data[3]"=w1018:u8, "Data[4]"=w1017:u8)  [unwired: 1 out]
                n480 = To Word Integer(number=w1020) -> (16bit integer=w1028:i16)
                n481 = To Word Integer(number=w1018) -> (16bit integer=w1024:i16)
                n482 = Rotate(1:w1028, 2:w1021) -> (0:w1027:i16)
                n483 = Rotate(1:w1024, 2:w1021) -> (0:w1023:i16)
                n484 = Add(x=w1027, y=w1019) -> (x+y=w1026:i16)
                n485 = Add(x=w1023, y=w1017) -> (x+y=w1022:i16)
                n486 = Divide(x=w1026, y=w1015) -> (x/y=w1013:dbl)
                "Iqnow" <- w1013
                n487 = Divide(x=w1022, y=w1015) -> (x/y=w1012:dbl)
                "Idnow" <- w1012
                n488 = Build Array(w1013, w1012) -> (w1014:dbl[])
              }
              frame 53 {
                w1038 = i16 1024
                w1037 = 8
                n489 = Array To Cluster(array=w1036) -> (cluster=w1042:T14)
                n490 = Unbundle By Name(w1042) -> ("Data[1]"=w1035:u8, "Data[2]"=w1034:u8, "Data[3]"=w1033:u8, "Data[4]"=w1032:u8)  [unwired: 1 out]
                n491 = To Word Integer(number=w1035) -> (16bit integer=w1045:i16)
                n492 = To Word Integer(number=w1033) -> (16bit integer=w1041:i16)
                n493 = Rotate(1:w1045, 2:w1037) -> (0:w1044:i16)
                n494 = Rotate(1:w1041, 2:w1037) -> (0:w1040:i16)
                n495 = Add(x=w1044, y=w1034) -> (x+y=w1043:i16)
                n496 = Add(x=w1040, y=w1032) -> (x+y=w1039:i16)
                n497 = Divide(x=w1043, y=w1038) -> (x/y=w1030:dbl)
                "Uq" <- w1030
                n498 = Divide(x=w1039, y=w1038) -> (x/y=w1029:dbl)
                "Ud" <- w1029
                n499 = Build Array(w1030, w1029) -> (w1031:dbl[])
              }
              frame 54 {
                w1055 = i16 1024
                w1054 = 8
                n500 = Array To Cluster(array=w1049) -> (cluster=w1059:T14)
                n501 = Unbundle By Name(w1059) -> ("Data[1]"=w1053:u8, "Data[2]"=w1052:u8, "Data[3]"=w1051:u8, "Data[4]"=w1050:u8)  [unwired: 1 out]
                n502 = To Word Integer(number=w1053) -> (16bit integer=w1062:i16)
                n503 = To Word Integer(number=w1051) -> (16bit integer=w1058:i16)
                n504 = Rotate(1:w1062, 2:w1054) -> (0:w1061:i16)
                n505 = Rotate(1:w1058, 2:w1054) -> (0:w1057:i16)
                n506 = Add(x=w1061, y=w1052) -> (x+y=w1060:i16)
                n507 = Add(x=w1057, y=w1050) -> (x+y=w1056:i16)
                n508 = Divide(x=w1060, y=w1055) -> (x/y=w1047:dbl)
                "Ualfa" <- w1047
                n509 = Divide(x=w1056, y=w1055) -> (x/y=w1046:dbl)
                "Ubate" <- w1046
                n510 = Build Array(w1047, w1046) -> (w1048:dbl[])
              }
              frame 55 {
                w1076 = u16 0
                w1075 = 8
                n511 = Array To Cluster(array=w1074) -> (cluster=w1083:T14)
                n512 = Unbundle By Name(w1083) -> ("Data[1]"=w1068:u8, "Data[2]"=w1069:u8, "Data[3]"=w1070:u8, "Data[4]"=w1071:u8, "Data[5]"=w1072:u8, "Data[6]"=w1073:u8, "Data[7]"=w1064:u8)  [unwired: 1 out]
                "sector" <- w1064
                n513 = To Word Integer(number=w1068) -> (16bit integer=w1086:i16)
                n514 = To Word Integer(number=w1070) -> (16bit integer=w1082:i16)
                n515 = To Word Integer(number=w1072) -> (16bit integer=w1079:i16)
                n516 = Rotate(1:w1086, 2:w1075) -> (0:w1085:i16)
                n517 = Rotate(1:w1082, 2:w1075) -> (0:w1081:i16)
                n518 = Rotate(1:w1079, 2:w1075) -> (0:w1078:i16)
                n519 = Add(x=w1085, y=w1069) -> (x+y=w1084:i16)
                n520 = Add(x=w1081, y=w1071) -> (x+y=w1080:i16)
                n521 = Add(x=w1078, y=w1073) -> (x+y=w1077:i16)
                n522 = Subtract ("减")(x=w1084, y=w1076) -> (x-y=w1067:u16)
                "PWM1" <- w1067
                n523 = Subtract ("减")(x=w1080, y=w1076) -> (x-y=w1066:u16)
                "PWM2" <- w1066
                n524 = Subtract ("减")(x=w1077, y=w1076) -> (x-y=w1065:u16)
                "PWM3" <- w1065
                n525 = Build Array(w1067, w1066, w1065, w1064) -> (w1063:u16[])
              }
              frame 56 {
                n526 = Array Subset(array=w1093, index=1, length=4) -> (w1090:u8[])
                n527 = Type Cast(type=2097152, x=w1090) -> (*(type *) &x=w1088:i32)
                "Sin" <- w1088
                "Cosin" <- w1088
                n528 = Build Array(w1088, w1088) -> (w1087:i32[])
              }
              frame 58 {
                n529 = Array To Cluster(array=w1096) -> (cluster=w1101:T14)
                n530 = Unbundle By Name(w1101) -> ("Data[1]"=w1099:u8, "Data[2]"=w1098:u8)  [unwired: 1 out]
                n531 = Join Numbers(hi=w1099, lo=w1098) -> ((hi.lo)=w1100:u16)
                n532 = To Unsigned Word Integer(number=w1100) -> (unsigned 16bit integer=w1097:u16)
                n533 = Multiply(x=w1097, y=0.0054931640625) -> (x*y=w1095:dbl)
                n534 = property on="机械角度" class="DigNum (严格)"("Value"=w1095) -> ()  [unwired: 2 in, 2 out]
              }
              frame 59 {
                n535 = Array To Cluster(array=w1103) -> (cluster=w1109:T14)
                n536 = Unbundle By Name(w1109) -> ("Data[1]"=w1107:u8, "Data[2]"=w1106:u8)  [unwired: 1 out]
                n537 = Join Numbers(hi=w1107, lo=w1106) -> ((hi.lo)=w1108:u16)
                n538 = To Word Integer(number=w1108) -> (16bit integer=w1105:i16)
                n539 = Divide(x=w1105, y=i16 1) -> (x/y=w1102:dbl)
                n540 = property on="转速" class="DigNum (严格)"("Value"=w1102) -> ()  [unwired: 2 in, 2 out]
              }
              frame 60 {
                n541 = Array To Cluster(array=w1111) -> (cluster=w1117:T14)
                n542 = Unbundle By Name(w1117) -> ("Data[1]"=w1115:u8, "Data[2]"=w1114:u8)  [unwired: 1 out]
                n543 = Join Numbers(hi=w1115, lo=w1114) -> ((hi.lo)=w1116:u16)
                n544 = To Word Integer(number=w1116) -> (16bit integer=w1113:i16)
                n545 = Divide(x=w1113, y=i16 256) -> (x/y=w1110:dbl)
                n546 = property on="Iqnow" class="DigNum (严格)"("Value"=w1110) -> ()  [unwired: 2 in, 2 out]
              }
              frame 61 {
                n547 = Array To Cluster(array=w1121) -> (cluster=w1125:T14)
                n548 = Unbundle By Name(w1125) -> ("Data[1]"=w1123:u8, "Data[2]"=w1122:u8)  [unwired: 1 out]
                n549 = Join Numbers(hi=w1123, lo=w1122) -> ((hi.lo)=w1124:u16)
                n550 = To Word Integer(number=w1124) -> (16bit integer=w1120:i16)
                n551 = Divide(x=w1120, y=i16 4) -> (x/y=→"温度":dbl)
              }
              frame 64 {
                n552 = Array To Cluster(array=w1127) -> (cluster=w1132:T14)
                n553 = Unbundle By Name(w1132) -> ("Data[1]"=w1128:u8, "Data[2]"=w1129:u8)  [unwired: 1 out]
                n554 = To Unsigned Word Integer(number=w1128) -> (unsigned 16bit integer=w1135:u16)
                n555 = Rotate(1:w1135, 2:8) -> (0:w1134:u16)
                n556 = Add ("加")(x=w1134, y=w1129) -> (x+y=w1133:u16)
                n557 = Divide(x=w1133, y=u16 256) -> (x/y=→"设定位置_回":dbl)
              }
              frame 65 {
                n558 = Array To Cluster(array=w1140) -> (cluster=w1141:T14)
                n559 = Unbundle By Name(w1141) -> ("Data[1]"=w1138:u8, "Data[2]"=w1137:u8)  [unwired: 1 out]
                n560 = Join Numbers(hi=w1138, lo=w1137) -> ((hi.lo)=w1139:u16)
                n561 = To Word Integer(number=w1139) -> (16bit integer=→"设定速度_回":i16)
              }
              frame 66 {
                n562 = Array To Cluster(array=w1143) -> (cluster=w1148:T14)
                n563 = Unbundle By Name(w1148) -> ("Data[1]"=w1144:u8, "Data[2]"=w1145:u8)  [unwired: 1 out]
                n564 = To Word Integer(number=w1144) -> (16bit integer=w1151:i16)
                n565 = Rotate(1:w1151, 2:8) -> (0:w1150:i16)
                n566 = Add ("加")(x=w1150, y=w1145) -> (x+y=w1149:i16)
                n567 = Divide(x=w1149, y=u16 256) -> (x/y=→"设定电流_回":dbl)
              }
              frame 81 {
                n568 = Array To Cluster(array=w1153) -> (cluster=w1158:T14)
                n569 = Unbundle By Name(w1158) -> ("Data[1]"=w1154:u8, "Data[2]"=w1155:u8)  [unwired: 1 out]
                n570 = To Unsigned Word Integer(number=w1154) -> (unsigned 16bit integer=w1161:u16)
                n571 = Rotate(1:w1161, 2:8) -> (0:w1160:u16)
                n572 = Add ("加")(x=w1160, y=w1155) -> (x+y=w1159:u16)
                n573 = Divide(x=w1159, y=u16 256) -> (x/y=→"电流环KP_回":dbl)
              }
              frame 82 {
                n574 = Array To Cluster(array=w1163) -> (cluster=w1168:T14)
                n575 = Unbundle By Name(w1168) -> ("Data[1]"=w1164:u8, "Data[2]"=w1165:u8)  [unwired: 1 out]
                n576 = To Unsigned Word Integer(number=w1164) -> (unsigned 16bit integer=w1171:u16)
                n577 = Rotate(1:w1171, 2:8) -> (0:w1170:u16)
                n578 = Add ("加")(x=w1170, y=w1165) -> (x+y=w1169:u16)
                n579 = Divide(x=w1169, y=u16 256) -> (x/y=→"电流环KI_回":dbl)
              }
              frame 83 {
                n580 = Array To Cluster(array=w1173) -> (cluster=w1178:T14)
                n581 = Unbundle By Name(w1178) -> ("Data[1]"=w1174:u8, "Data[2]"=w1175:u8)  [unwired: 1 out]
                n582 = To Unsigned Word Integer(number=w1174) -> (unsigned 16bit integer=w1181:u16)
                n583 = Rotate(1:w1181, 2:8) -> (0:w1180:u16)
                n584 = Add ("加")(x=w1180, y=w1175) -> (x+y=w1179:u16)
                n585 = Divide(x=w1179, y=u16 256) -> (x/y=→"速度环KP_回":dbl)
              }
              frame 84 {
                n586 = Array To Cluster(array=w1183) -> (cluster=w1188:T14)
                n587 = Unbundle By Name(w1188) -> ("Data[1]"=w1184:u8, "Data[2]"=w1185:u8)  [unwired: 1 out]
                n588 = To Unsigned Word Integer(number=w1184) -> (unsigned 16bit integer=w1191:u16)
                n589 = Rotate(1:w1191, 2:8) -> (0:w1190:u16)
                n590 = Add ("加")(x=w1190, y=w1185) -> (x+y=w1189:u16)
                n591 = Divide(x=w1189, y=u16 256) -> (x/y=→"速度环KI_回":dbl)
              }
              frame 85 {
                n592 = Array To Cluster(array=w1193) -> (cluster=w1198:T14)
                n593 = Unbundle By Name(w1198) -> ("Data[1]"=w1194:u8, "Data[2]"=w1195:u8)  [unwired: 1 out]
                n594 = To Unsigned Word Integer(number=w1194) -> (unsigned 16bit integer=w1201:u16)
                n595 = Rotate(1:w1201, 2:8) -> (0:w1200:u16)
                n596 = Add ("加")(x=w1200, y=w1195) -> (x+y=w1199:u16)
                n597 = Divide(x=w1199, y=u16 8) -> (x/y=→"加速度_回":dbl)
              }
              frame 90 {
                n598 = Array To Cluster(array=w1206) -> (cluster=w1207:T14)
                n599 = Unbundle By Name(w1207) -> ("Data[1]"=w1204:u8, "Data[2]"=w1203:u8)  [unwired: 1 out]
                n600 = Join Numbers(hi=w1204, lo=w1203) -> ((hi.lo)=w1205:u16)
                n601 = To Unsigned Word Integer(number=w1205) -> (unsigned 16bit integer=→"AI_K0_回":u16)
              }
              frame 91 {
                n602 = Array To Cluster(array=w1209) -> (cluster=w1213:T14)
                n603 = Unbundle By Name(w1213) -> ("Data[1]"=w1211:u8, "Data[2]"=w1210:u8)  [unwired: 1 out]
                n604 = Join Numbers(hi=w1211, lo=w1210) -> ((hi.lo)=w1212:u16)
                n605 = To Unsigned Word Integer(number=w1212) -> (unsigned 16bit integer=→"BI_K0_回":u16)
              }
              frame 92 {
                n606 = Array To Cluster(array=w1215) -> (cluster=w1219:T14)
                n607 = Unbundle By Name(w1219) -> ("Data[1]"=w1217:u8, "Data[2]"=w1216:u8)  [unwired: 1 out]
                n608 = Join Numbers(hi=w1217, lo=w1216) -> ((hi.lo)=w1218:u16)
                n609 = To Unsigned Word Integer(number=w1218) -> (unsigned 16bit integer=→"CI_K0_回":u16)
              }
            }
            n610 = case shown="真" w881 {
              tunnel: w880 -> [_ w891]
              tunnel: w879 -> [_ w889]
              frame False {
              }
              frame True {
                n611 = Array Size(array=w889) -> (size(s)=w890:i32)
                n612 = Open/Create/Replace File(file path (use dialog)=w891, operation (0:open)=T11."open or create") -> (refnum out=w899:refnum<file>, error out=w888:errorcluster)  [unwired: 4 in, 1 out]
                n613 = for {
                  N: w890 -> [_]
                  shift-right: [w907] -> w896
                  shift-left: "" -> [w904]
                  tunnel: w889 -> [w902]
                  i -> [w903]
                  # "浮点文本存储"
                  # "2-14"
                  n614 = Index Array(array=w902, index=w903) -> (element=w901:dbl)
                  n615 = Number To Fractional String(number=w901) -> (F-format string=w906:string)  [unwired: 3 in]
                  n616 = Concatenate Strings(w904, w906, "\t") -> (w907:string)
                }
                n617 = Set File Position(refnum=w899, from (0:start)=u16 1, error in=w888) -> (refnum out=w898:refnum<file>, error out=w887:errorcluster)  [unwired: 1 in]
                n618 = Concatenate Strings(w896, "\r") -> (w894:string)
                n619 = Write to Text File(file (use dialog)=w898, text=w894, error in=w887) -> (refnum out=w897:refnum<file>, error out=w886:errorcluster)  [unwired: 1 in, 1 out]
                n620 = Close File(refnum=w897, error in=w886) -> (error out=w885:errorcluster)  [unwired: 1 out]
                n621 = call <vilib>:"Clear Errors.vi"("error in (no error)"=w885) -> ()  [unwired: 6 in, 1 out]
              }
            }
          }
        }
      }
      frame True {
      }
    }
  }
  n622 = while "接收线程" {
    tunnel: w9 -> [w1223]
    shift-right: [w1221] -> _
    shift-left: u32 0 ("RecvCnt") -> [w1222]
    stop <- "RcvEnable" continue-if-true
    n623 = local read "Open"() -> (w1224:bool)
    n624 = case shown="真" w1224 {
      tunnel: w1223 -> [_ w1231]
      tunnel: w1222 -> [w1226 w1230]
      tunnel: [w1226 w1229] -> w1221
      frame False {
        # "CAN未打开，延时50ms"
        n625 = Wait (ms)(milliseconds to wait=u32 50 ("等待时间（毫秒）")) -> ()  [unwired: 1 out]
      }
      frame True {
        n626 = local read "DevType"() -> (w1235:T5)
        n627 = local read "Channel"() -> (w1228:T4)
        n628 = call "VCI_Receive.vi"("CANIndex"=w1228, "DevIndex"=u32 0, "DevType"=w1235) -> ("Recieve"=w1232:T6[])  [unwired: 3 in, 5 out]
        n629 = Empty Array?(array=w1232) -> (empty?=w1233:bool)
        n630 = case shown="假" w1233 {
          tunnel: w1231 -> [w1242 _]
          tunnel: w1232 -> [w1237 _]
          tunnel: [w1241 _] -> _
          tunnel: w1230 -> [w1239 w1254]
          tunnel: [w1238 w1254] -> w1229
          tunnel: w1228 -> [w1240 _]
          frame False {
            n631 = Array Size(array=w1237) -> (size(s)=w1236:i32)
            n632 = for {
              N: w1236 -> [_]
              tunnel: w1242 -> [w1253]
              tunnel: [w1251] -> w1241 mode=indexing
              tunnel: w1237 -> [w1246]
              tunnel: w1240 -> [w1250]
              shift-right: [w1247] -> w1238
              shift-left: w1239 -> [w1248]
              i -> [w1244]
              n633 = Array Subset(array=w1246, index=w1244, length=1) -> (w1245:T6[])
              n634 = Increment(x=w1248) -> (x+1=w1247:u32)
              n635 = call "Demo_MakeDispBuff.vi"("Channel"=w1250, "Type"=enum16{"接收", "发送"}."接收", "OBJs"=w1245) -> ("Buffer"=w1252:T7)
              n636 = Enqueue Element(queue=w1253, element=w1252) -> (error out=w1251:errorcluster)  [unwired: 1 in, 3 out]
            }
            "RecvCnt" <- w1238
          }
          frame True {
          }
        }
      }
    }
  }
  n637 = control-ref of="本应用程序"() -> (w6:refnum<vi>)
  n638 = invoke class="VI" method="FP.Close"(error in=w4) -> (error out=w3:errorcluster)  [unwired: 2 in, 2 out]
  n639 = property class="App"(reference=w6) -> ("App.Kind"=w5:T16)  [unwired: 1 in, 2 out]
  n640 = case shown="\"Development System\"" w5 {
    tunnel: w3 -> [_ _]
    frame "invalid app kind", Default {
      n641 = Quit LabVIEW() -> ()  [unwired: 1 out]
    }
    frame "Development System" {
    }
  }
